vi "FGV_REPORTS_records_display.vi"(7 "options":T1, 8 "error_in":errorcluster, 11 "input":variant) -> (0 "error_out":errorcluster, 3 "output":variant)   [LabVIEW 2019]
uses:
  FGV_REPORTS_records_display.ctl
  REPORTS_references.ctl
  REPORTS_all_info.ctl
  MAIN/REPORTS/GEAR/typedef/REPORT_GEAR_all_info.ctl
  MAIN/REPORTS/GEAR/typedef/REPORT_GEAR_header_data_display.ctl
  MAIN/REPORTS/GEAR/typedef/REPORT_GEAR_statuses.ctl
  MAIN/REPORTS/DATES/typedef/REPORT_DATES_all_info.ctl
  MAIN/REPORTS/DATES/typedef/REPORT_DATES_statuses.ctl
  MAIN/REPORTS/PRODUCTION_BATCH/typedef/REPORT_PBATCH_all_info.ctl
  MAIN/REPORTS/OPERATION/typedef/REPORT_OPRTN_all_info.ctl
  MAIN/REPORTS/CONFIG_HISTORY/typedef/REPORT_CFG_all_info.ctl
  MAIN/REPORTS/CONFIG_HISTORY/typedef/REPORT_CFG_types.ctl
  MAIN/REPORTS/AUDIT/typedef/REPORT_AUDIT_all_info.ctl
  MAIN/REPORTS/OK_NOK_COUNT/typedef/REPORT_OKNOK_all_info.ctl
  MAIN/REPORTS/REWORKS/typedef/REPORT_REWORKS_all_info.ctl
  MAIN/REPORTS/PACE/typedef/REPORT_PACE_all_info.ctl
  MAIN/REPORTS/CUSTOMER_BATCH/typedef/REPORT_CBATCH_all_info.ctl
  MAIN/REPORTS/GEAR_COMPONENTS/typedef/REPORT_CMPNT_all_info.ctl
  MAIN/REPORTS/DATES/typedef/REPORT_DATES_filters.ctl
  MAIN/REPORTS/PRODUCTION_BATCH/typedef/REPORT_PBATCH_filters.ctl
  MAIN/REPORTS/OPERATION/typedef/REPORT_OPRTN_filters.ctl
  MAIN/REPORTS/CONFIG_HISTORY/typedef/REPORT_CFG_filters.ctl
  MAIN/REPORTS/AUDIT/typedef/REPORT_AUDIT_filters.ctl
  MAIN/REPORTS/REWORKS/typedef/REPORT_REWORKS_stations.ctl
  MAIN/REPORTS/REPORT_page_change.ctl
  _misc/AULocalize/SubVIs/Get Localized Phrase Compact Interface 0D.vi
  _misc/AULocalize/SubVIs/Get Localized Phrase Compact Interface 1D.vi
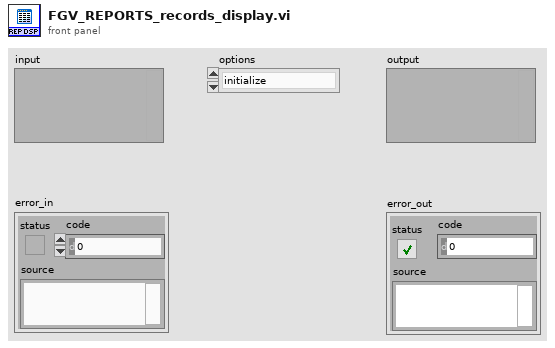
[diagram p1: front panel]
types:
  T1 = typedef "FGV_REPORTS_records_display.ctl" = enum16{"initialize", "GEAR_set_serial", "GEAR_set_header", "GEAR_set_operations", "GEAR_set_results", "GEAR_set_batches", "GEAR_get_serial", "GEAR_get_operation_IDs", "GEAR_toggle_results", "GEAR_show_all_results", "GEAR_hide_all_results", "GEAR_display", "GEAR_filter", "GEAR_restore", "GEAR_clear", "GEAR_get_all_info", "DATES_set_dates", "DATES_set_gears", "DATES_display", "DATES_filter", "DATES_first_page", "DATES_previous_page", "DATES_next_page", "DATES_last_page", "DATES_restore", "DATES_clear", "DATES_get_all_info", "PBATCH_set_batch_no", "PBATCH_set_gears", "PBATCH_display", "PBATCH_filter", "PBATCH_first_page", "PBATCH_previous_page", "PBATCH_next_page", "PBATCH_last_page", "PBATCH_restore", "PBATCH_clear", "PBATCH_get_all_info", "OPRTN_set_OP", "OPRTN_set_dates", "OPRTN_set_gears", "OPRTN_set_hidden_columns", "OPRTN_display", "OPRTN_filter", "OPRTN_filter_no_page_reset", "OPRTN_first_page", "OPRTN_previous_page", "OPRTN_next_page", "OPRTN_last_page", "OPRTN_restore", "OPRTN_clear", "OPRTN_get_all_info", "CFG_set_type", "CFG_set_dates", "CFG_set_records", "CFG_display", "CFG_filter", "CFG_first_page", "CFG_previous_page", "CFG_next_page", "CFG_last_page", "CFG_restore", "CFG_clear", "CFG_get_all_info", "AUDIT_set_dates", "AUDIT_set_records", "AUDIT_display", "AUDIT_filter", "AUDIT_first_page", "AUDIT_previous_page", "AUDIT_next_page", "AUDIT_last_page", "AUDIT_restore", "AUDIT_clear", "AUDIT_get_all_info", "OKNOK_set_dates", "OKNOK_set_records", "OKNOK_display", "OKNOK_restore", "OKNOK_clear", "OKNOK_get_all_info", "REWORKS_set_dates", "REWORKS_set_from_to", "REWORKS_set_records", "REWORKS_display", "REWORKS_filter", "REWORKS_first_page", "REWORKS_previous_page", "REWORKS_next_page", "REWORKS_last_page", "REWORKS_restore", "REWORKS_clear", "REWORKS_get_all_info", "PACE_set_dates", "PACE_set_limits", "PACE_set_records", "PACE_display", "PACE_restore", "PACE_clear", "PACE_get_all_info", "CBATCH_set_code", "CBATCH_set_records", "CBATCH_display", "CBATCH_filter", "CBATCH_first_page", "CBATCH_previous_page", "CBATCH_next_page", "CBATCH_last_page", "CBATCH_restore", "CBATCH_clear", "CBATCH_get_all_info", "CMPNT_set_serial", "CMPNT_set_records", "CMPNT_display", "CMPNT_first_page", "CMPNT_previous_page", "CMPNT_next_page", "CMPNT_last_page", "CMPNT_restore", "CMPNT_clear", "CMPNT_get_all_info", "clear"}
  T2 = typedef "REPORTS_all_info.ctl" = cluster{"REPORT_GEAR_all_info":T3, "REPORT_DATES_all_info":T6, "REPORT_PBATCH_all_info":T8, "REPORT_OPRTN_all_info":T9, "REPORT_CFG_all_info":T10, "REPORT_AUDIT_all_info":T12, "REPORT_OKNOK_all_info":T13, "REPORT_REWORKS_all_info":T14, "REPORT_PACE_all_info":T15, "REPORT_CBATCH_all_info":T16, "REPORT_CMPNT_all_info":T17, "REPORTS_references":T18}
  T3 = typedef "REPORT_GEAR_all_info.ctl" = cluster{"serial":string, "filter_OP":string, "REPORT_GEAR_header":T4, "operations":string[][], "operation_statuses":T5[], "results":string[][], "result_statuses":T5[], "batches":string[][], "batch_statuses":T5[], "column_headers":string[], "displayed_rows":string[][], "displayed_statuses":T5[], "column_widths":i16[]}
  T4 = typedef "REPORT_GEAR_header_data_display.ctl" = cluster{"ID":string, "creation_time":string, "last_station":string, "last_status":string, "pinion_serial":string, "batch_code":string}
  T5 = typedef "REPORT_GEAR_statuses.ctl" = enum16{"OP_OK_hide", "OP_OK_show", "OP_NOK_hide", "OP_NOK_show", "OP_interrupted_hide", "OP_interrupted_show", "OP_in_operation_hide", "OP_in_operation_show", "OP_unexpected_hide", "OP_unexpected_show", "RE_REAL_OK", "RE_REAL_NOK", "RE_STRING", "RE_sub_header", "RE_no_data", "RE_unexpected", "BA_sub_header", "BA_data", "BA_no_data"}
  T6 = typedef "REPORT_DATES_all_info.ctl" = cluster{"date_start":string, "date_end":string, "time_start":string, "time_end":string, "filter_last_OP":string, "filter_last_status":string, "gears":string[][], "gears_statuses":T7[], "column_headers":string[], "displayed_rows":string[][], "displayed_statuses":T7[], "column_widths":i16[], "active_page":i32}
  T7 = typedef "REPORT_DATES_statuses.ctl" = enum16{"GEAR_OK", "GEAR_NOK", "GEAR_interrupted", "GEAR_in_operation", "GEAR_unexpected"}
  T8 = typedef "REPORT_PBATCH_all_info.ctl" = cluster{"batch_no":string, "filter_last_OP":string, "filter_last_status":string, "gears":string[][], "gears_statuses":T7[], "column_headers":string[], "displayed_rows":string[][], "displayed_statuses":T7[], "column_widths":i16[], "active_page":i32}
  T9 = typedef "REPORT_OPRTN_all_info.ctl" = cluster{"OP":string, "date_start":string, "date_end":string, "time_start":string, "time_end":string, "filter_last_status":string, "no_of_static_columns":i32, "operations":string[][], "operations_statuses":T7[], "column_headers":string[], "archivisation_description":string[][], "displayed_rows":string[][], "displayed_statuses":T7[], "column_widths":i16[], "hidden_columns":i32[], "active_page":i32}
  T10 = typedef "REPORT_CFG_all_info.ctl" = cluster{"type":T11, "date_start":string, "date_end":string, "time_start":string, "time_end":string, "filter_OP":string, "records":string[][], "column_headers":string[], "displayed_rows":string[][], "column_widths":i16[], "active_page":i32}
  T11 = typedef "REPORT_CFG_types.ctl" = enum16{"REFERENCE", "ARCHIVISATION", "USERS"}
  T12 = typedef "REPORT_AUDIT_all_info.ctl" = cluster{"date_start":string, "date_end":string, "time_start":string, "time_end":string, "filter_OP":string, "filter_status":string, "records":string[][], "record_statuses":T7[], "column_headers":string[], "displayed_rows":string[][], "displayed_statuses":T7[], "column_widths":i16[], "active_page":i32}
  T13 = typedef "REPORT_OKNOK_all_info.ctl" = cluster{"date_start":string, "date_end":string, "time_start":string, "time_end":string, "records":string[][], "column_headers":string[], "column_widths":i16[]}
  T14 = typedef "REPORT_REWORKS_all_info.ctl" = cluster{"date_start":string, "date_end":string, "time_start":string, "time_end":string, "from_OP":string, "to_OP":string, "records":string[][], "record_statuses":T7[], "column_headers":string[], "displayed_rows":string[][], "displayed_statuses":T7[], "column_widths":i16[], "active_page":i32}
  T15 = typedef "REPORT_PACE_all_info.ctl" = cluster{"date_start":string, "date_end":string, "time_start":string, "time_end":string, "low_limit":u16, "high_limit":u16, "records":string[][], "column_headers":string[], "column_widths":i16[]}
  T16 = typedef "REPORT_CBATCH_all_info.ctl" = cluster{"batch_code":string, "records":string[][], "record_statuses":T7[], "column_headers":string[], "displayed_rows":string[][], "displayed_statuses":T7[], "column_widths":i16[], "active_page":i32}
  T17 = typedef "REPORT_CMPNT_all_info.ctl" = cluster{"gear_serial":string, "records":string[][], "column_headers":string[], "displayed_rows":string[][], "column_widths":i16[], "active_page":i32}
  T18 = typedef "REPORTS_references.ctl" = cluster{"front_panel_reference":refnum<vi>, "SQL_listbox_reference":refnum<vi>, "REPORT_page_first":refnum<vi>, "REPORT_page_previous":refnum<vi>, "REPORT_page_next":refnum<vi>, "REPORT_page_last":refnum<vi>, "REPORT_page_counter":refnum<vi>, "REPORT_GEAR_serial":refnum<vi>, "REPORT_GEAR_serial_display":refnum<vi>, "REPORT_GEAR_station":refnum<vi>, "REPORT_GEAR_header_data_display":refnum<vi>, "REPORT_DATES_start":refnum<vi>, "REPORT_DATES_end":refnum<vi>, "REPORT_DATES_time_start":refnum<vi>, "REPORT_DATES_time_end":refnum<vi>, "REPORT_DATES_order_selection":refnum<vi>, "REPORT_DATES_last_OP":refnum<vi>, "REPORT_DATES_last_status":refnum<vi>, "REPORT_PBATCH_batch_no":refnum<vi>, "REPORT_PBATCH_order_selection":refnum<vi>, "REPORT_PBATCH_last_op":refnum<vi>, "REPORT_PBATCH_last_status":refnum<vi>, "REPORT_OPRTN_operation":refnum<vi>, "REPORT_OPRTN_start":refnum<vi>, "REPORT_OPRTN_end":refnum<vi>, "REPORT_OPRTN_time_start":refnum<vi>, "REPORT_OPRTN_time_end":refnum<vi>, "REPORT_OPRTN_order_selection":refnum<vi>, "REPORT_OPRTN_last_status":refnum<vi>, "REPORT_CFG_type":refnum<vi>, "REPORT_CFG_start":refnum<vi>, "REPORT_CFG_end":refnum<vi>, "REPORT_CFG_time_start":refnum<vi>, "REPORT_CFG_time_end":refnum<vi>, "REPORT_CFG_order_selection":refnum<vi>, "REPORT_CFG_op_filter":refnum<vi>, "REPORT_AUDIT_start":refnum<vi>, "REPORT_AUDIT_end":refnum<vi>, "REPORT_AUDIT_time_start":refnum<vi>, "REPORT_AUDIT_time_end":refnum<vi>, "REPORT_AUDIT_order_selection":refnum<vi>, "REPORT_AUDIT_op_filter":refnum<vi>, "REPORT_AUDIT_status_filter":refnum<vi>, "REPORT_OKNOK_start":refnum<vi>, "REPORT_OKNOK_end":refnum<vi>, "REPORT_OKNOK_time_start":refnum<vi>, "REPORT_OKNOK_time_end":refnum<vi>, "REPORT_REWORKS_start":refnum<vi>, "REPORT_REWORKS_end":refnum<vi>, "REPORT_REWORKS_time_start":refnum<vi>, "REPORT_REWORKS_time_end":refnum<vi>, "REPORT_REWORKS_from_OP":refnum<vi>, "REPORT_REWORKS_to_OP":refnum<vi>, "REPORT_REWORKS_order_selection":refnum<vi>, "REPORT_PACE_start":refnum<vi>, "REPORT_PACE_end":refnum<vi>, "REPORT_PACE_time_start":refnum<vi>, "REPORT_PACE_time_end":refnum<vi>, "REPORT_PACE_low_limit":refnum<vi>, "REPORT_PACE_high_limit":refnum<vi>, "REPORT_CBATCH_batch_code":refnum<vi>, "REPORT_CBATCH_order_selection":refnum<vi>, "REPORT_CMPNT_gear_serial":refnum<vi>}
  T19 = typedef "REPORT_DATES_filters.ctl" = cluster{"order_selection":enum32{"old_to_new", "new_to_old"}, "last_OP":string, "last_status":string}
  T20 = typedef "REPORT_page_change.ctl" = enum16{"first", "previous", "next", "last"}
  T21 = typedef "REPORT_PBATCH_filters.ctl" = cluster{"order_selection":enum32{"old_to_new", "new_to_old"}, "last_OP":string, "last_status":string}
  T22 = typedef "REPORT_OPRTN_filters.ctl" = cluster{"order_selection":enum32{"old_to_new", "new_to_old"}, "last_status":string}
  T23 = typedef "REPORT_CFG_filters.ctl" = cluster{"order_selection":enum32{"old_to_new", "new_to_old"}, "OP":string}
  T24 = typedef "REPORT_AUDIT_filters.ctl" = cluster{"order_selection":enum32{"old_to_new", "new_to_old"}, "OP_filter":string, "status_filter":string}
  T25 = typedef "REPORT_REWORKS_stations.ctl" = u16
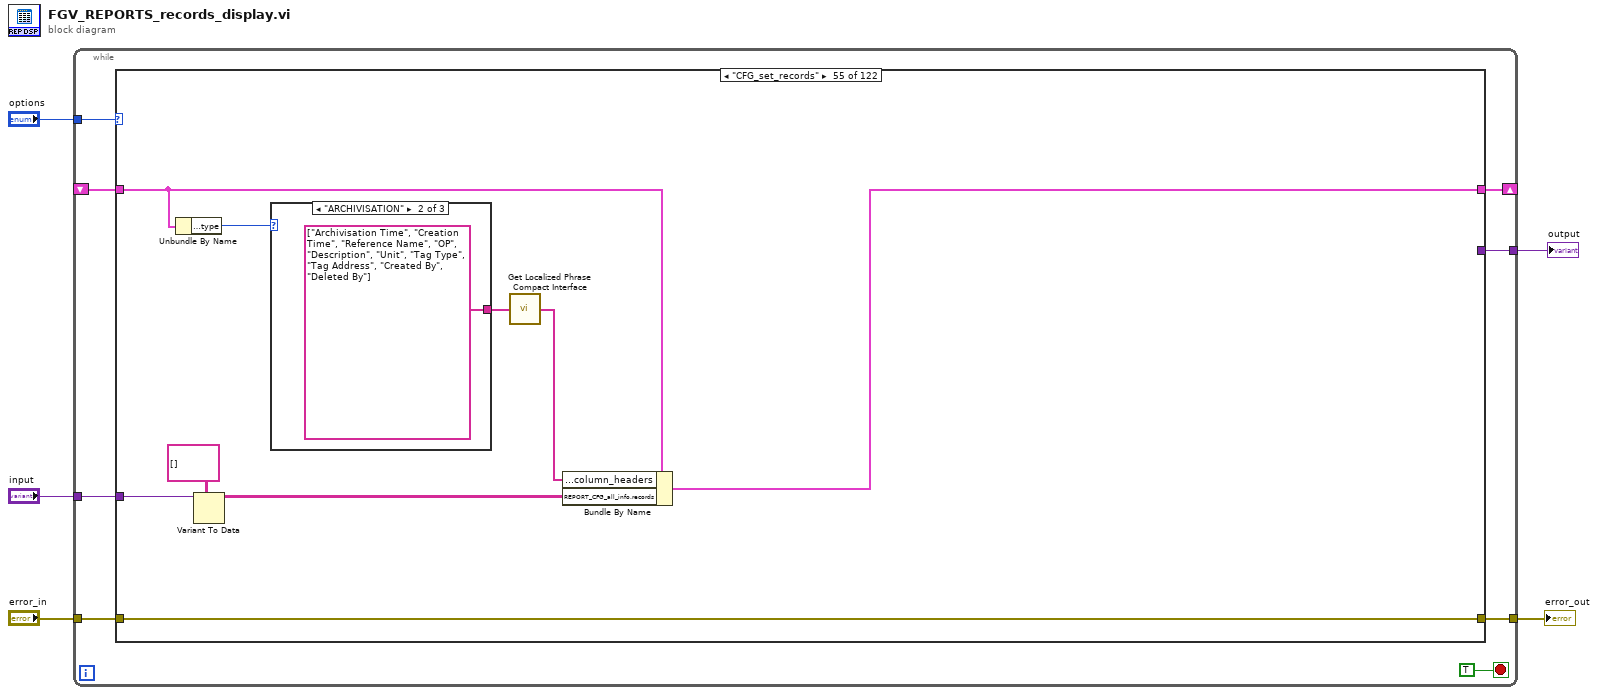
[diagram p0: block diagram]
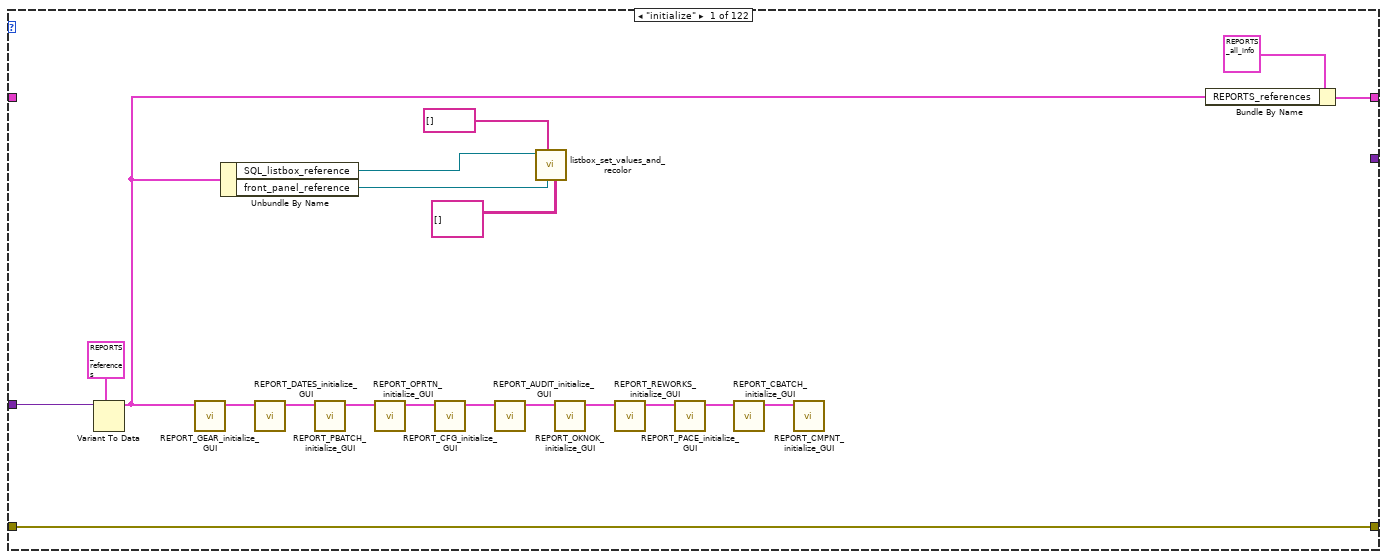
[diagram p2: hidden frame]
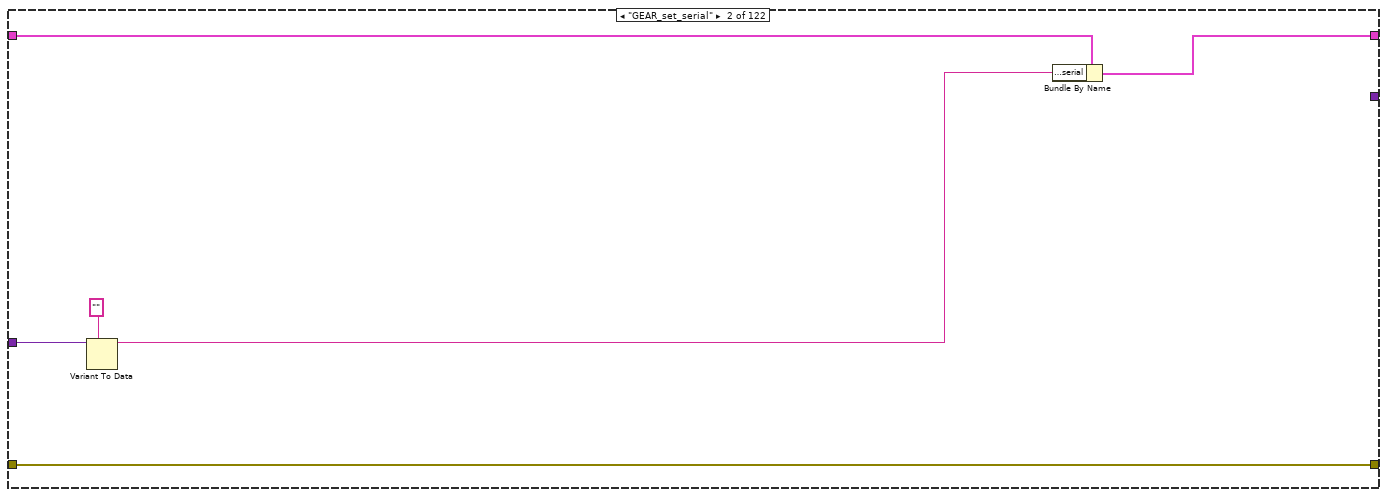
[diagram p3: hidden frame]
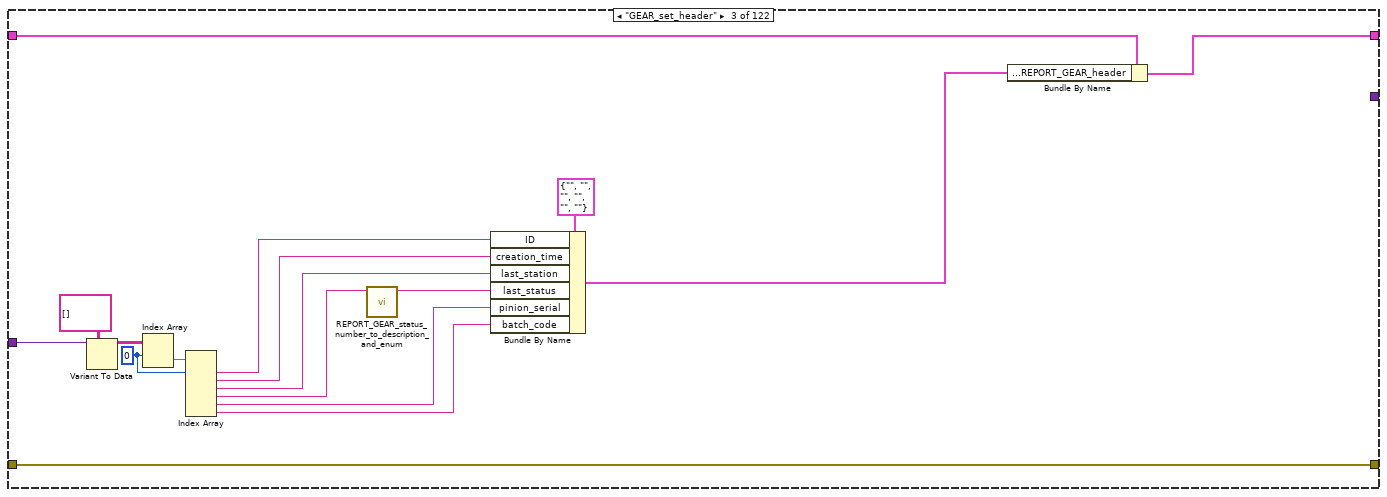
[diagram p4: hidden frame]
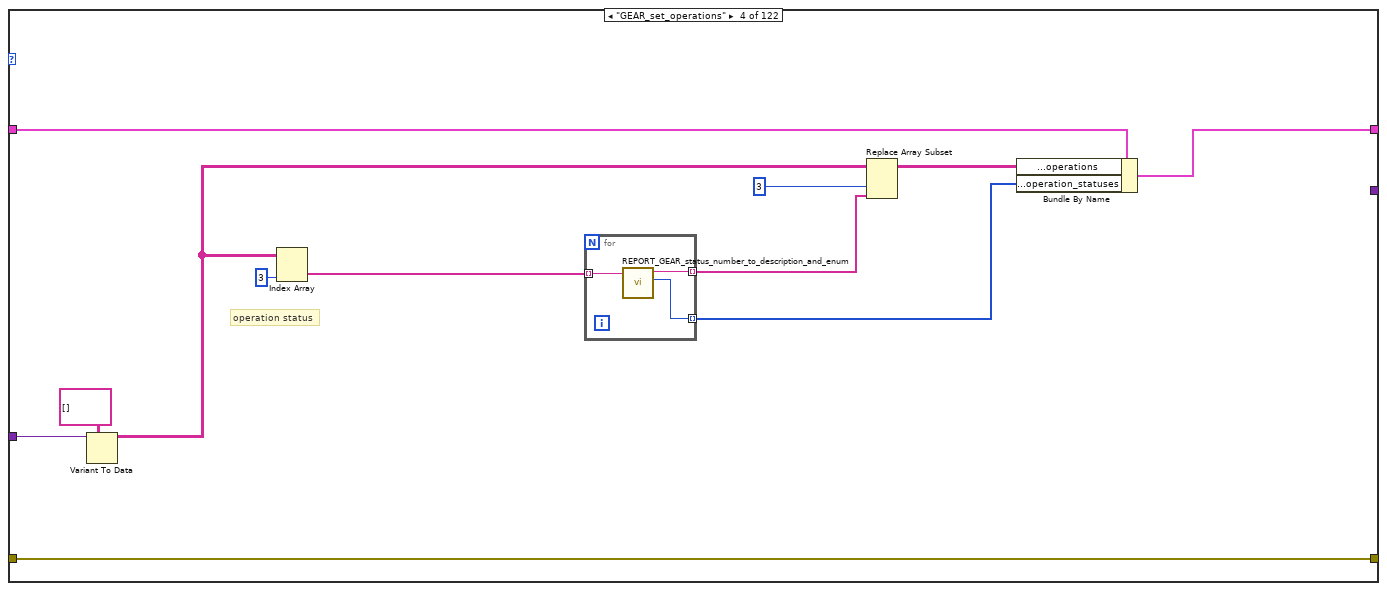
[diagram p5: hidden frame]
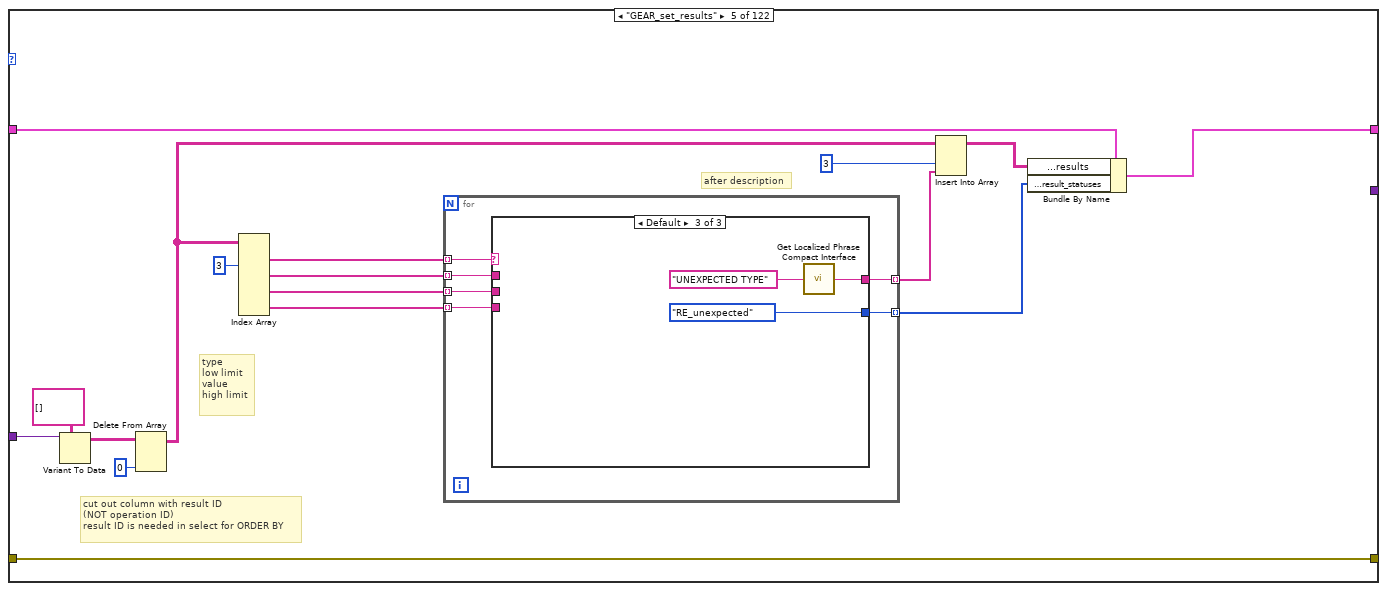
[diagram p6: hidden frame]
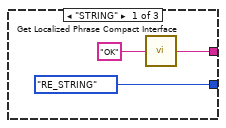
[diagram p7: hidden frame]
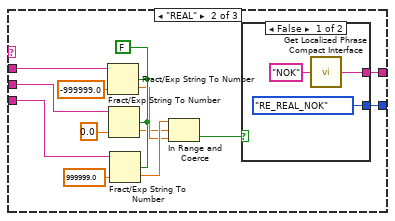
[diagram p8: hidden frame]
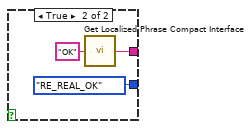
[diagram p9: hidden frame]
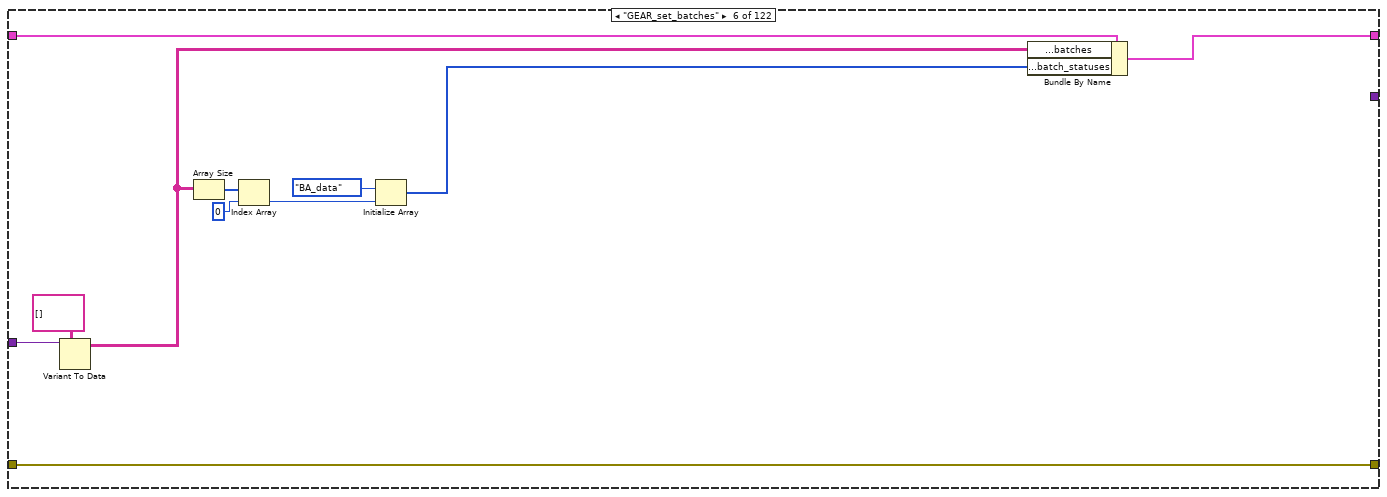
[diagram p10: hidden frame]
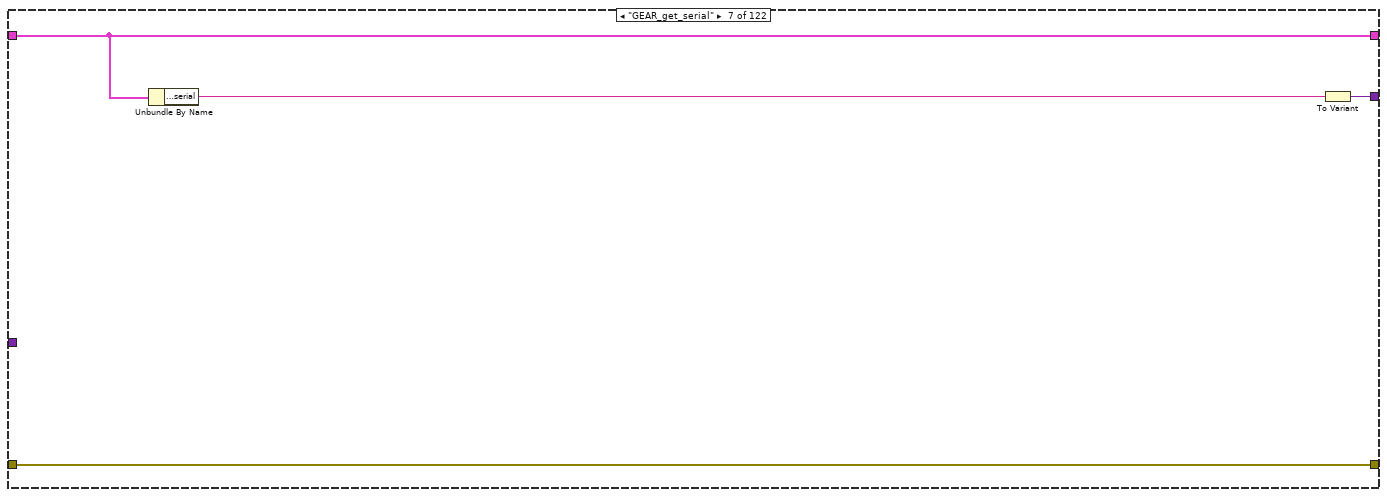
[diagram p11: hidden frame]
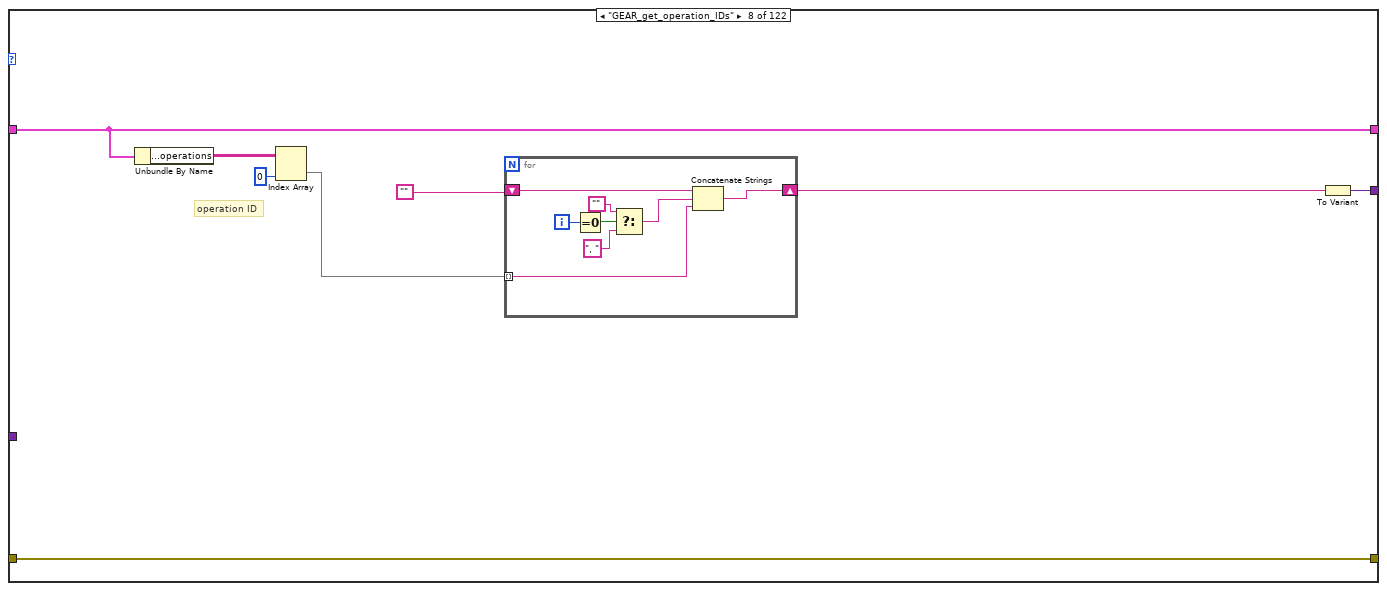
[diagram p12: hidden frame]
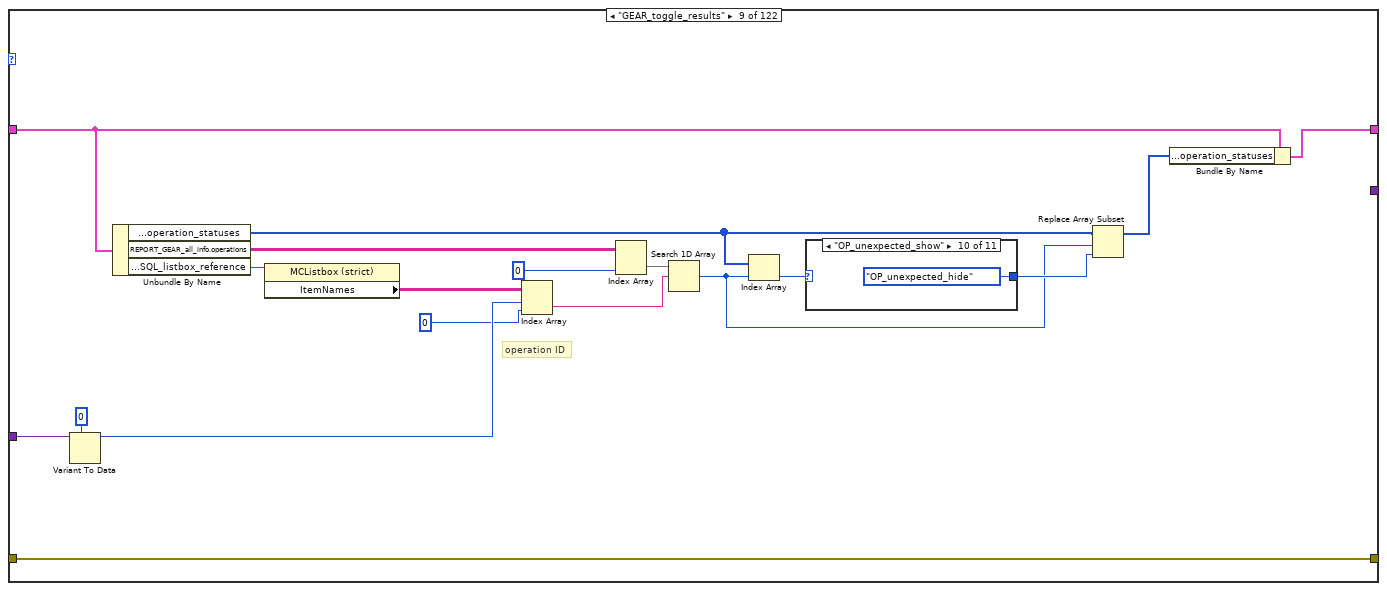
[diagram p13: hidden frame]
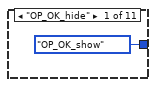
[diagram p14: hidden frame]
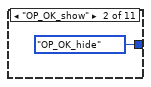
[diagram p15: hidden frame]
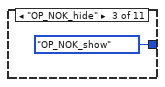
[diagram p16: hidden frame]
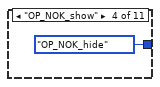
[diagram p17: hidden frame]
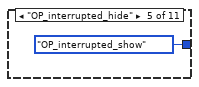
[diagram p18: hidden frame]
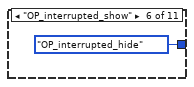
[diagram p19: hidden frame]
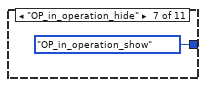
[diagram p20: hidden frame]
diagram:
  n1 = while {
    tunnel: "options" -> [w12]
    tunnel: [w11] -> w5
    tunnel: "error_in" -> [w10]
    shift-right: [w9] -> _
    shift-left: _ -> [w8]
    tunnel: "input" -> [w7]
    tunnel: [w6] -> w1
    stop <- TRUE stop-if-true
    n2 = case shown="\"CFG_set_records\"" w12 {
      tunnel: [w33 w39 w56 w68 w88 w130 w134 w142 w168 w184 w197 w212 w218 w220 w229 w233 w244 w256 w269 w275 w279 w283 w287 w291 w293 w302 w306 w312 w324 w337 w343 w347 w351 w355 w359 w361 w370 w374 w380 w391 w410 w425 w434 w441 w448 w452 w456 w460 w464 w466 w475 w479 w485 w496 w505 w516 w522 w526 w530 w534 w538 w540 w549 w553 w564 w576 w589 w595 w599 w603 w607 w611 w613 w622 w626 w637 w643 w648 w650 w659 w663 w674 w683 w695 w706 w712 w716 w720 w724 w728 w730 w739 w743 w754 w762 w768 w773 w775 w784 w788 w794 w806 w817 w823 w827 w831 w835 w839 w841 w850 w854 w860 w866 w871 w875 w879 w883 w887 w889 w898 w902 w911] -> w11
      tunnel: w10 -> [w33 w39 w56 w68 w88 w130 w134 w142 w168 w184 w197 w212 w218 w220 w229 w233 w244 w256 w269 w275 w279 w283 w287 w291 w293 w302 w306 w312 w324 w337 w343 w347 w351 w355 w359 w361 w370 w374 w380 w391 w410 w425 w434 w441 w448 w452 w456 w460 w464 w466 w475 w479 w485 w496 w505 w516 w522 w526 w530 w534 w538 w540 w549 w553 w564 w576 w589 w595 w599 w603 w607 w611 w613 w622 w626 w637 w643 w648 w650 w659 w663 w674 w683 w695 w706 w712 w716 w720 w724 w728 w730 w739 w743 w754 w762 w768 w773 w775 w784 w788 w794 w806 w817 w823 w827 w831 w835 w839 w841 w850 w854 w860 w866 w871 w875 w879 w883 w887 w889 w898 w902 w911]
      tunnel: [w25 w38 w55 w67 w87 w129 w132 w140 w152 w182 w195 w207 w217 w219 w228 w232 w238 w255 w262 w274 w277 w281 w285 w289 w292 w301 w305 w311 w323 w330 w340 w345 w349 w353 w357 w360 w369 w373 w379 w385 w409 w422 w428 w438 w445 w450 w454 w458 w462 w465 w474 w478 w484 w490 w503 w510 w519 w524 w528 w532 w536 w539 w548 w552 w558 w575 w582 w594 w597 w601 w605 w609 w612 w621 w625 w631 w642 w645 w649 w658 w662 w668 w682 w694 w700 w711 w714 w718 w722 w726 w729 w738 w742 w748 w761 w767 w770 w774 w783 w787 w791 w805 w812 w822 w825 w829 w833 w837 w840 w849 w853 w857 w865 w868 w873 w877 w881 w885 w888 w897 w901 w903] -> w9
      tunnel: w8 -> [_ w36 w53 w65 w85 w127 w132 w140 w153 w183 w196 w208 w216 w219 w227 w232 w239 w253 w267 w273 w278 w282 w286 w290 w292 w300 w305 w309 w321 w335 w341 w346 w350 w354 w358 w360 w368 w373 w377 w386 w407 w423 w433 w439 w446 w451 w455 w459 w463 w465 w473 w478 w482 w491 w500 w515 w520 w525 w529 w533 w537 w539 w547 w552 w559 w573 w587 w593 w598 w602 w606 w610 w612 w620 w625 w632 w640 w646 w649 w657 w662 w669 w680 w692 w704 w710 w715 w719 w723 w727 w729 w737 w742 w749 w759 w765 w771 w774 w782 w787 w792 w803 w815 w821 w826 w830 w834 w838 w840 w848 w853 w858 w863 w869 w874 w878 w882 w886 w888 w896 w901 w908]
      tunnel: w7 -> [w29 w37 w54 w66 w86 w128 _ _ w166 _ _ _ w215 _ _ _ w243 w254 w266 w272 _ _ _ _ _ _ _ w310 w322 w334 w342 _ _ _ _ _ _ _ w378 w390 w408 w424 w432 w440 w447 _ _ _ _ _ _ _ w483 w495 w504 w514 w521 _ _ _ _ _ _ _ w563 w574 w586 w592 _ _ _ _ _ _ _ w636 w641 _ _ _ _ w673 w681 w693 w703 w709 _ _ _ _ _ _ _ w753 w760 w766 _ _ _ _ w793 w804 w814 w820 _ _ _ _ _ _ _ w859 w864 _ _ _ _ _ _ _ _ _]
      tunnel: [_ _ _ _ _ _ w133 w141 _ _ _ _ _ _ _ w230 _ _ _ _ _ _ _ _ _ _ w303 _ _ _ _ _ _ _ _ _ _ w371 _ _ _ _ _ _ _ _ _ _ _ _ _ w476 _ _ _ _ _ _ _ _ _ _ _ w550 _ _ _ _ _ _ _ _ _ _ w623 _ _ _ _ _ w660 _ _ _ _ _ _ _ _ _ _ _ w740 _ _ _ _ _ _ w785 _ _ _ _ _ _ _ _ _ _ w851 _ _ _ _ _ _ _ _ _ w899 _] -> w6
      frame "initialize" {
        n3 = Variant To Data(type=T18 {"front_panel_reference"=refnum, "SQL_listbox_reference"=refnum, "REPORT_page_first"=refnum, "REPORT_page_previous"=refnum, "REPORT_page_next"=refnum, "REPORT_page_last"=refnum, "REPORT_page_counter"=refnum, "REPORT_GEAR_serial"=refnum, "REPORT_GEAR_serial_display"=refnum, "REPORT_GEAR_station"=refnum, "REPORT_GEAR_header_data_display"=refnum, "REPORT_DATES_start"=refnum, "REPORT_DATES_end"=refnum, "REPORT_DATES_time_start"=refnum, "REPORT_DATES_time_end"=refnum, "REPORT_DATES_order_selection"=refnum, "REPORT_DATES_last_OP"=refnum, "REPORT_DATES_last_status"=refnum, "REPORT_PBATCH_batch_no"=refnum, "REPORT_PBATCH_order_selection"=refnum, "REPORT_PBATCH_last_op"=refnum, "REPORT_PBATCH_last_status"=refnum, "REPORT_OPRTN_operation"=refnum, "REPORT_OPRTN_start"=refnum, "REPORT_OPRTN_end"=refnum, "REPORT_OPRTN_time_start"=refnum, "REPORT_OPRTN_time_end"=refnum, "REPORT_OPRTN_order_selection"=refnum, "REPORT_OPRTN_last_status"=refnum, "REPORT_CFG_type"=refnum, "REPORT_CFG_start"=refnum, "REPORT_CFG_end"=refnum, "REPORT_CFG_time_start"=refnum, "REPORT_CFG_time_end"=refnum, "REPORT_CFG_order_selection"=refnum, "REPORT_CFG_op_filter"=refnum, "REPORT_AUDIT_start"=refnum, "REPORT_AUDIT_end"=refnum, "REPORT_AUDIT_time_start"=refnum, "REPORT_AUDIT_time_end"=refnum, "REPORT_AUDIT_order_selection"=refnum, "REPORT_AUDIT_op_filter"=refnum, "REPORT_AUDIT_status_filter"=refnum, "REPORT_OKNOK_start"=refnum, "REPORT_OKNOK_end"=refnum, "REPORT_OKNOK_time_start"=refnum, "REPORT_OKNOK_time_end"=refnum, "REPORT_REWORKS_start"=refnum, "REPORT_REWORKS_end"=refnum, "REPORT_REWORKS_time_start"=refnum, "REPORT_REWORKS_time_end"=refnum, "REPORT_REWORKS_from_OP"=refnum, "REPORT_REWORKS_to_OP"=refnum, "REPORT_REWORKS_order_selection"=refnum, "REPORT_PACE_start"=refnum, "REPORT_PACE_end"=refnum, "REPORT_PACE_time_start"=refnum, "REPORT_PACE_time_end"=refnum, "REPORT_PACE_low_limit"=refnum, "REPORT_PACE_high_limit"=refnum, "REPORT_CBATCH_batch_code"=refnum, "REPORT_CBATCH_order_selection"=refnum, "REPORT_CMPNT_gear_serial"=refnum} ("REPORTS_references"), Variant=w29) -> (data=w24:T18)  [unwired: 1 in, 1 out]
        n4 = call "REPORT_GEAR_initialize_GUI.vi"("REPORTS_references_in"=w24) -> ("REPORTS_references_out"=w23:T18)  [unwired: 10 in]
        n5 = Unbundle By Name(w24) -> ("SQL_listbox_reference"=w27:refnum<vi>, "front_panel_reference"=w28:refnum<vi>)
        n6 = call "REPORT_DATES_initialize_GUI.vi"("REPORTS_references_in"=w23) -> ("REPORTS_references_out"=w22:T18)  [unwired: 10 in]
        n7 = call "REPORT_PBATCH_initialize_GUI.vi"("REPORTS_references_in"=w22) -> ("REPORTS_references_out"=w21:T18)  [unwired: 10 in]
        n8 = call "REPORT_OPRTN_initialize_GUI.vi"("REPORTS_references_in"=w21) -> ("REPORTS_references_out"=w20:T18)  [unwired: 10 in]
        n9 = call "REPORT_CFG_initialize_GUI.vi"("REPORTS_references_in"=w20) -> ("REPORTS_references_out"=w19:T18)  [unwired: 10 in]
        n10 = call "REPORT_AUDIT_initialize_GUI.vi"("REPORTS_references_in"=w19) -> ("REPORTS_references_out"=w18:T18)  [unwired: 10 in]
        n11 = call "listbox_set_values_and_recolor.vi"("item_names"=string[][] [], "front_panel_reference"=w28, "column_names"=string[] [], "multicolumn_listbox_reference_in"=w27) -> ()  [unwired: 6 in, 2 out]
        n12 = call "REPORT_OKNOK_initialize_GUI.vi"("REPORTS_references_in"=w18) -> ("REPORTS_references_out"=w17:T18)  [unwired: 10 in]
        n13 = call "REPORT_REWORKS_initialize_GUI.vi"("REPORTS_references_in"=w17) -> ("REPORTS_references_out"=w16:T18)  [unwired: 10 in]
        n14 = call "REPORT_PACE_initialize_GUI.vi"("REPORTS_references_in"=w16) -> ("REPORTS_references_out"=w15:T18)  [unwired: 10 in]
        n15 = call "REPORT_CBATCH_initialize_GUI.vi"("REPORTS_references_in"=w15) -> ("REPORTS_references_out"=w14:T18)  [unwired: 10 in]
        n16 = call "REPORT_CMPNT_initialize_GUI.vi"("REPORTS_references_in"=w14) -> ()  [unwired: 10 in, 1 out]
        n17 = Bundle By Name(cluster=T2 {"REPORT_GEAR_all_info"={"serial"="", "filter_OP"="", "REPORT_GEAR_header"={"ID"="", "creation_time"="", "last_station"="", "last_status"="", "pinion_serial"="", "batch_code"=""}, "operations"=[], "operation_statuses"=[], "results"=[], "result_statuses"=[], "batches"=[], "batch_statuses"=[], "column_headers"=[], "displayed_rows"=[], "displayed_statuses"=[], "column_widths"=[]}, "REPORT_DATES_all_info"={"date_start"="", "date_end"="", "time_start"="", "time_end"="", "filter_last_OP"="", "filter_last_status"="", "gears"=[], "gears_statuses"=[], "column_headers"=[], "displayed_rows"=[], "displayed_statuses"=[], "column_widths"=[], "active_page"=0}, "REPORT_PBATCH_all_info"={"batch_no"="", "filter_last_OP"="", "filter_last_status"="", "gears"=[], "gears_statuses"=[], "column_headers"=[], "displayed_rows"=[], "displayed_statuses"=[], "column_widths"=[], "active_page"=0}, "REPORT_OPRTN_all_info"={"OP"="", "date_start"="", "date_end"="", "time_start"="", "time_end"="", "filter_last_status"="", "no_of_static_columns"=0, "operations"=[], "operations_statuses"=[], "column_headers"=[], "archivisation_description"=[], "displayed_rows"=[], "displayed_statuses"=[], "column_widths"=[], "hidden_columns"=[], "active_page"=0}, "REPORT_CFG_all_info"={"type"=enum."REFERENCE", "date_start"="", "date_end"="", "time_start"="", "time_end"="", "filter_OP"="", "records"=[], "column_headers"=[], "displayed_rows"=[], "column_widths"=[], "active_page"=0}, "REPORT_AUDIT_all_info"={"date_start"="", "date_end"="", "time_start"="", "time_end"="", "filter_OP"="", "filter_status"="", "records"=[], "record_statuses"=[], "column_headers"=[], "displayed_rows"=[], "displayed_statuses"=[], "column_widths"=[], "active_page"=0}, "REPORT_OKNOK_all_info"={"date_start"="", "date_end"="", "time_start"="", "time_end"="", "records"=[], "column_headers"=[], "column_widths"=[]}, "REPORT_REWORKS_all_info"={"date_start"="", "date_end"="", "time_start"="", "time_end"="", "from_OP"="", "to_OP"="", "records"=[], "record_statuses"=[], "column_headers"=[], "displayed_rows"=[], "displayed_statuses"=[], "column_widths"=[], "active_page"=0}, "REPORT_PACE_all_info"={"date_start"="", "date_end"="", "time_start"="", "time_end"="", "low_limit"=0, "high_limit"=0, "records"=[], "column_headers"=[], "column_widths"=[]}, "REPORT_CBATCH_all_info"={"batch_code"="", "records"=[], "record_statuses"=[], "column_headers"=[], "displayed_rows"=[], "displayed_statuses"=[], "column_widths"=[], "active_page"=0}, "REPORT_CMPNT_all_info"={"gear_serial"="", "records"=[], "column_headers"=[], "displayed_rows"=[], "column_widths"=[], "active_page"=0}, "REPORTS_references"={"front_panel_reference"=refnum, "SQL_listbox_reference"=refnum, "REPORT_page_first"=refnum, "REPORT_page_previous"=refnum, "REPORT_page_next"=refnum, "REPORT_page_last"=refnum, "REPORT_page_counter"=refnum, "REPORT_GEAR_serial"=refnum, "REPORT_GEAR_serial_display"=refnum, "REPORT_GEAR_station"=refnum, "REPORT_GEAR_header_data_display"=refnum, "REPORT_DATES_start"=refnum, "REPORT_DATES_end"=refnum, "REPORT_DATES_time_start"=refnum, "REPORT_DATES_time_end"=refnum, "REPORT_DATES_order_selection"=refnum, "REPORT_DATES_last_OP"=refnum, "REPORT_DATES_last_status"=refnum, "REPORT_PBATCH_batch_no"=refnum, "REPORT_PBATCH_order_selection"=refnum, "REPORT_PBATCH_last_op"=refnum, "REPORT_PBATCH_last_status"=refnum, "REPORT_OPRTN_operation"=refnum, "REPORT_OPRTN_start"=refnum, "REPORT_OPRTN_end"=refnum, "REPORT_OPRTN_time_start"=refnum, "REPORT_OPRTN_time_end"=refnum, "REPORT_OPRTN_order_selection"=refnum, "REPORT_OPRTN_last_status"=refnum, "REPORT_CFG_type"=refnum, "REPORT_CFG_start"=refnum, "REPORT_CFG_end"=refnum, "REPORT_CFG_time_start"=refnum, "REPORT_CFG_time_end"=refnum, "REPORT_CFG_order_selection"=refnum, "REPORT_CFG_op_filter"=refnum, "REPORT_AUDIT_start"=refnum, "REPORT_AUDIT_end"=refnum, "REPORT_AUDIT_time_start"=refnum, "REPORT_AUDIT_time_end"=refnum, "REPORT_AUDIT_order_selection"=refnum, "REPORT_AUDIT_op_filter"=refnum, "REPORT_AUDIT_status_filter"=refnum, "REPORT_OKNOK_start"=refnum, "REPORT_OKNOK_end"=refnum, "REPORT_OKNOK_time_start"=refnum, "REPORT_OKNOK_time_end"=refnum, "REPORT_REWORKS_start"=refnum, "REPORT_REWORKS_end"=refnum, "REPORT_REWORKS_time_start"=refnum, "REPORT_REWORKS_time_end"=refnum, "REPORT_REWORKS_from_OP"=refnum, "REPORT_REWORKS_to_OP"=refnum, "REPORT_REWORKS_order_selection"=refnum, "REPORT_PACE_start"=refnum, "REPORT_PACE_end"=refnum, "REPORT_PACE_time_start"=refnum, "REPORT_PACE_time_end"=refnum, "REPORT_PACE_low_limit"=refnum, "REPORT_PACE_high_limit"=refnum, "REPORT_CBATCH_batch_code"=refnum, "REPORT_CBATCH_order_selection"=refnum, "REPORT_CMPNT_gear_serial"=refnum}} ("REPORT_all_info"), "REPORTS_references"=w24) -> (w25:T2)
      }
      frame "GEAR_set_serial" {
        n18 = Variant To Data(type="", Variant=w37) -> (data=w34:string)  [unwired: 1 in, 1 out]
        n19 = Bundle By Name(cluster=w36, "REPORT_GEAR_all_info.serial"=w34) -> (w38:T2)
      }
      frame "GEAR_set_header" {
        w47 = 0 ("index (row)")
        n20 = Variant To Data(type=string[][] [], Variant=w54) -> (data=w49:string[][])  [unwired: 1 in, 1 out]
        n21 = Index Array(array=w49, index (row)=w47) -> (element=w48:string[])  [unwired: 1 in]
        n22 = Index Array(array=w48, index #1=w47) -> (element #1=w45:string, element #2=w46:string, element #3=w44:string, element #4=w42:string, element #5=w43:string, element #6=w40:string)  [unwired: 5 in]
        n23 = call "REPORT_GEAR_status_number_to_description_and_enum.vi"("status_nmb"=w42) -> ("status_description"=w41:string)  [unwired: 9 in, 1 out]
        n24 = Bundle By Name(cluster=T4 {"ID"="", "creation_time"="", "last_station"="", "last_status"="", "pinion_serial"="", "batch_code"=""} ("REPORT_GEAR_header_data_display"), "ID"=w45, "creation_time"=w46, "last_station"=w44, "last_status"=w41, "pinion_serial"=w43, "batch_code"=w40) -> (w50:T4)
        n25 = Bundle By Name(cluster=w53, "REPORT_GEAR_all_info.REPORT_GEAR_header"=w50) -> (w55:T2)
      }
      frame "GEAR_set_operations" {
        # "operation status"
        n26 = Variant To Data(type=string[][] [], Variant=w66) -> (data=w60:string[][])  [unwired: 1 in, 1 out]
        n27 = Index Array(array=w60, index (col)=3 ("disabled index (col)")) -> (element=w62:string[])  [unwired: 1 in]
        n28 = for {
          tunnel: w62 -> [w71] mode=indexing
          tunnel: [w70] -> w61 mode=indexing
          tunnel: [w69] -> w57 mode=indexing
          n29 = call "REPORT_GEAR_status_number_to_description_and_enum.vi"("status_nmb"=w71) -> ("status_enum"=w70:T5, "status_description"=w69:string)  [unwired: 9 in]
        }
        n30 = Replace Array Subset(array=w60, new element=w57, index (col)=3 ("disabled index (col)")) -> (w58:string[][])  [unwired: 1 in]
        n31 = Bundle By Name(cluster=w65, "REPORT_GEAR_all_info.operations"=w58, "REPORT_GEAR_all_info.operation_statuses"=w61) -> (w67:T2)
      }
      frame "GEAR_set_results" {
        # "after description"
        # "cut out column with result ID\n(NOT operation ID)\nresult ID is needed in select for ORDER BY"
        # "type\nlow limit\nvalue\nhigh limit"
        n32 = Variant To Data(type=string[][] [], Variant=w86) -> (data=w75:string[][])  [unwired: 1 in, 1 out]
        n33 = Delete From Array(array=w75, index (col)=0 ("disabled index (col)")) -> (array with subset deleted=w74:string[][])  [unwired: 2 in, 1 out]
        n34 = Index Array(array=w74, index (col) #1=3 ("disabled index (col)")) -> (element #1=w78:string[], element #2=w83:string[], element #3=w81:string[], element #4=w80:string[])  [unwired: 7 in]
        n35 = for {
          tunnel: w83 -> [w91] mode=indexing
          tunnel: [w94] -> w82 mode=indexing
          tunnel: [w93] -> w76 mode=indexing
          tunnel: w81 -> [w90] mode=indexing
          tunnel: w80 -> [w89] mode=indexing
          tunnel: w78 -> [w92] mode=indexing
          n36 = case shown="Default" w92 {
            tunnel: [REPORT_GEAR_statuses."RE_STRING" ("REPORT_GEAR_statuses") w110 REPORT_GEAR_statuses."RE_unexpected" ("REPORT_GEAR_statuses")] -> w94
            tunnel: [w95 w109 w117] -> w93
            tunnel: w91 -> [_ w108 _]
            tunnel: w90 -> [_ w106 _]
            tunnel: w89 -> [_ w105 _]
            frame "STRING" {
              n37 = call-poly "Get Localized Phrase Compact Interface.vi"("Key"="OK") -> ("Translated Phrase"=w95:string)
            }
            frame "REAL" {
              w107 = FALSE ("use system decimal point (T)")
              n38 = Fract/Exp String To Number(use system decimal point (T)=w107, string=w108, default (0 dbl)=sgl -999999.0 ("default (0 DBL)")) -> (number=w103:sgl)  [unwired: 1 in, 1 out]
              n39 = Fract/Exp String To Number(use system decimal point (T)=w107, string=w106, default (0 dbl)=sgl 0.0 ("default (0 DBL)")) -> (number=w102:sgl)  [unwired: 1 in, 1 out]
              n40 = Fract/Exp String To Number(use system decimal point (T)=w107, string=w105, default (0 dbl)=sgl 999999.0 ("default (0 DBL)")) -> (number=w104:sgl)  [unwired: 1 in, 1 out]
              n41 = In Range and Coerce(upper limit=w104, x=w102, lower limit=w103) -> (In Range?=w101:bool)  [unwired: 1 out]
              n42 = case shown="False" w101 {
                tunnel: [REPORT_GEAR_statuses."RE_REAL_NOK" ("REPORT_GEAR_statuses") REPORT_GEAR_statuses."RE_REAL_OK" ("REPORT_GEAR_statuses")] -> w110
                tunnel: [w111 w114] -> w109
                frame False {
                  n43 = call-poly "Get Localized Phrase Compact Interface.vi"("Key"="NOK") -> ("Translated Phrase"=w111:string)
                }
                frame True {
                  n44 = call-poly "Get Localized Phrase Compact Interface.vi"("Key"="OK") -> ("Translated Phrase"=w114:string)
                }
              }
            }
            frame Default {
              n45 = call-poly "Get Localized Phrase Compact Interface.vi"("Key"="UNEXPECTED TYPE") -> ("Translated Phrase"=w117:string)
            }
          }
        }
        n46 = Insert Into Array(array=w74, index (col)=3 ("disabled index (col)"), new element=w76) -> (w77:string[][])  [unwired: 1 in]
        n47 = Bundle By Name(cluster=w85, "REPORT_GEAR_all_info.results"=w77, "REPORT_GEAR_all_info.result_statuses"=w82) -> (w87:T2)
      }
      frame "GEAR_set_batches" {
        n48 = Variant To Data(type=string[][] [], Variant=w128) -> (data=w124:string[][])  [unwired: 1 in, 1 out]
        n49 = Array Size(array=w124) -> (size(s)=w123:i32[])
        n50 = Index Array(array=w123, index=0) -> (element=w121:i32)
        n51 = Initialize Array(REPORT_GEAR_statuses."BA_data" ("REPORT_GEAR_statuses"), w121) -> (w120:T5[])
        n52 = Bundle By Name(cluster=w127, "REPORT_GEAR_all_info.batches"=w124, "REPORT_GEAR_all_info.batch_statuses"=w120) -> (w129:T2)
      }
      frame "GEAR_get_serial" {
        n53 = Unbundle By Name(w132) -> ("REPORT_GEAR_all_info.serial"=w131:string)
        n54 = To Variant(anything=w131) -> (Variant=w133:variant)
      }
      frame "GEAR_get_operation_IDs" {
        # "operation ID"
        n55 = Unbundle By Name(w140) -> ("REPORT_GEAR_all_info.operations"=w139:string[][])
        n56 = Index Array(array=w139, index (col)=0 ("disabled index (col)")) -> (element=w137:string[])  [unwired: 1 in]
        n57 = for {
          tunnel: w137 -> [w143] mode=indexing
          shift-right: [w146] -> w135
          shift-left: "" -> [w145]
          i -> [w147]
          n58 = Equal To 0?(x=w147) -> (x = 0?=w148:bool)
          n59 = Select(t="", s=w148, f=", ") -> (s? t:f=w144:string)
          n60 = Concatenate Strings(w145, w144, w143) -> (w146:string)
        }
        n61 = To Variant(anything=w135) -> (Variant=w141:variant)
      }
      frame "GEAR_toggle_results" {
        # "operation ID"
        n62 = Variant To Data(type=0 ("Row"), Variant=w166) -> (data=w163:i32)  [unwired: 1 in, 1 out]
        n63 = Unbundle By Name(w153) -> ("REPORT_GEAR_all_info.operation_statuses"=w156:T5[], "REPORT_GEAR_all_info.operations"=w161:string[][], "REPORTS_references.SQL_listbox_reference"=w167:refnum<vi>)
        n64 = property class="MCListbox (strict)"(reference=w167) -> ("ItemNames"=w164:string[][])  [unwired: 1 in, 2 out]
        n65 = Index Array(array=w164, index (row)=w163, index (col)=0 ("disabled index (col)")) -> (element=w158:string)
        n66 = Index Array(array=w161, index (col)=0 ("disabled index (col)")) -> (element=w159:string[])  [unwired: 1 in]
        n67 = Search 1D Array(1D array=w159, element=w158) -> (index of element=w154:i32)  [unwired: 1 in]
        n68 = Index Array(array=w156, index=w154) -> (element=w157:T5)
        n69 = case shown="\"OP_unexpected_show\"" w157 {
          selector: w157 -> [_ _ _ _ _ _ _ _ _ _ w179]
          tunnel: [REPORT_GEAR_statuses."OP_OK_show" ("REPORT_GEAR_statuses") REPORT_GEAR_statuses."OP_OK_hide" ("REPORT_GEAR_statuses") REPORT_GEAR_statuses."OP_NOK_show" ("REPORT_GEAR_statuses") REPORT_GEAR_statuses."OP_NOK_hide" ("REPORT_GEAR_statuses") REPORT_GEAR_statuses."OP_interrupted_show" ("REPORT_GEAR_statuses") REPORT_GEAR_statuses."OP_interrupted_hide" ("REPORT_GEAR_statuses") REPORT_GEAR_statuses."OP_in_operation_show" ("REPORT_GEAR_statuses") REPORT_GEAR_statuses."OP_in_operation_hide" ("REPORT_GEAR_statuses") REPORT_GEAR_statuses."OP_unexpected_show" ("REPORT_GEAR_statuses") REPORT_GEAR_statuses."OP_unexpected_hide" ("REPORT_GEAR_statuses") w179] -> w155
          frame "OP_OK_hide" {
          }
          frame "OP_OK_show" {
          }
          frame "OP_NOK_hide" {
          }
          frame "OP_NOK_show" {
          }
          frame "OP_interrupted_hide" {
          }
          frame "OP_interrupted_show" {
          }
          frame "OP_in_operation_hide" {
          }
          frame "OP_in_operation_show" {
          }
          frame "OP_unexpected_hide" {
          }
          frame "OP_unexpected_show" {
          }
          frame Default {
          }
        }
        n70 = Replace Array Subset(array=w156, new element=w155, index=w154) -> (w151:T5[])
        n71 = Bundle By Name(cluster=w153, "REPORT_GEAR_all_info.operation_statuses"=w151) -> (w152:T2)
      }
      frame "GEAR_show_all_results" {
        n72 = Unbundle By Name(w183) -> ("REPORT_GEAR_all_info.operation_statuses"=w181:T5[])
        n73 = for {
          tunnel: w181 -> [w186] mode=indexing
          tunnel: [w185] -> w180 mode=indexing
          n74 = case shown="\"OP_OK_hide\"" w186 {
            selector: w186 -> [_ _ _ _ _ w192]
            tunnel: [REPORT_GEAR_statuses."OP_OK_show" ("REPORT_GEAR_statuses") REPORT_GEAR_statuses."OP_NOK_show" ("REPORT_GEAR_statuses") REPORT_GEAR_statuses."OP_interrupted_show" ("REPORT_GEAR_statuses") REPORT_GEAR_statuses."OP_in_operation_show" ("REPORT_GEAR_statuses") REPORT_GEAR_statuses."OP_unexpected_show" ("REPORT_GEAR_statuses") w192] -> w185
            frame "OP_OK_hide" {
            }
            frame "OP_NOK_hide" {
            }
            frame "OP_interrupted_hide" {
            }
            frame "OP_in_operation_hide" {
            }
            frame "OP_unexpected_hide" {
            }
            frame Default {
            }
          }
        }
        n75 = Bundle By Name(cluster=w183, "REPORT_GEAR_all_info.operation_statuses"=w180) -> (w182:T2)
      }
      frame "GEAR_hide_all_results" {
        n76 = Unbundle By Name(w196) -> ("REPORT_GEAR_all_info.operation_statuses"=w194:T5[])
        n77 = for {
          tunnel: w194 -> [w198] mode=indexing
          tunnel: [w199] -> w193 mode=indexing
          n78 = case shown="\"OP_unexpected_show\"" w198 {
            selector: w198 -> [_ _ _ _ _ w205]
            tunnel: [REPORT_GEAR_statuses."OP_OK_hide" ("REPORT_GEAR_statuses") REPORT_GEAR_statuses."OP_NOK_hide" ("REPORT_GEAR_statuses") REPORT_GEAR_statuses."OP_interrupted_hide" ("REPORT_GEAR_statuses") REPORT_GEAR_statuses."OP_in_operation_hide" ("REPORT_GEAR_statuses") REPORT_GEAR_statuses."OP_unexpected_hide" ("REPORT_GEAR_statuses") w205] -> w199
            frame "OP_OK_show" {
            }
            frame "OP_NOK_show" {
            }
            frame "OP_interrupted_show" {
            }
            frame "OP_in_operation_show" {
            }
            frame "OP_unexpected_show" {
            }
            frame Default {
            }
          }
        }
        n79 = Bundle By Name(cluster=w196, "REPORT_GEAR_all_info.operation_statuses"=w193) -> (w195:T2)
      }
      frame "GEAR_display" {
        n80 = Unbundle By Name(w208) -> ("REPORTS_references.REPORT_GEAR_header_data_display"=w211:refnum<vi>, "REPORT_GEAR_all_info.REPORT_GEAR_header"=w210:T4)
        n81 = call-poly "Get Localized Phrase Compact Interface.vi"("Key"=string[] ["ID", "Time", "OP", "Status", "Operator"] ("column_names")) -> ("Translated Phrase"=w206:string[])
        n82 = call "REPORT_GEAR_listbox_set_values_and_recolor.vi"("column_names"=w206, "REPORT_all_info_in"=w208) -> ("REPORT_all_info_out"=w207:T2)  [unwired: 8 in, 1 out]
        n83 = property class="Clust (strict)"(reference=w211, "Value"=w210) -> ()  [unwired: 1 in, 2 out]
      }
      frame "GEAR_filter" {
        n84 = Variant To Data(type="", Variant=w215) -> (data=w214:string)  [unwired: 1 in, 1 out]
        n85 = call "REPORT_GEAR_listbox_filter.vi"("OP"=w214, "REPORT_all_info_in"=w216) -> ("REPORT_all_info_out"=w217:T2)  [unwired: 8 in, 1 out]
      }
      frame "GEAR_restore" {
        n86 = call "REPORT_GEAR_listbox_restore.vi"("REPORT_all_info_in"=w219) -> ()  [unwired: 10 in, 1 out]
      }
      frame "GEAR_clear" {
        n87 = Unbundle By Name(w227) -> ("REPORTS_references"=w222:T18)
        n88 = call "REPORT_GEAR_initialize_GUI.vi"("REPORTS_references_in"=w222) -> ()  [unwired: 10 in, 1 out]
        n89 = Unbundle By Name(w222) -> ("SQL_listbox_reference"=w223:refnum<vi>, "front_panel_reference"=w224:refnum<vi>)
        n90 = call "listbox_set_values_and_recolor.vi"("item_names"=string[][] [], "front_panel_reference"=w224, "column_names"=string[] [], "multicolumn_listbox_reference_in"=w223) -> ()  [unwired: 6 in, 2 out]
        n91 = Bundle By Name(cluster=w227, "REPORT_GEAR_all_info"=T3 {"serial"="", "filter_OP"="", "REPORT_GEAR_header"={"ID"="", "creation_time"="", "last_station"="", "last_status"="", "pinion_serial"="", "batch_code"=""}, "operations"=[], "operation_statuses"=[], "results"=[], "result_statuses"=[], "batches"=[], "batch_statuses"=[], "column_headers"=[], "displayed_rows"=[], "displayed_statuses"=[], "column_widths"=[]}) -> (w228:T2)
      }
      frame "GEAR_get_all_info" {
        n92 = Unbundle By Name(w232) -> ("REPORT_GEAR_all_info"=w231:T3)
        n93 = To Variant(anything=w231) -> (Variant=w230:variant)
      }
      frame "DATES_set_dates" {
        n94 = Variant To Data(type=string[] [], Variant=w243) -> (data=w241:string[])  [unwired: 1 in, 1 out]
        n95 = Index Array(array=w241, index #1=0 ("index (row)")) -> (element #1=w236:string, element #2=w235:string, element #3=w234:string, element #4=w237:string)  [unwired: 3 in]
        n96 = Bundle By Name(cluster=w239, "REPORT_DATES_all_info.date_start"=w236, "REPORT_DATES_all_info.date_end"=w235, "REPORT_DATES_all_info.time_start"=w234, "REPORT_DATES_all_info.time_end"=w237) -> (w238:T2)
      }
      frame "DATES_set_gears" {
        # "gear last status"
        n97 = Variant To Data(type=string[][] [], Variant=w254) -> (data=w248:string[][])  [unwired: 1 in, 1 out]
        n98 = Index Array(array=w248, index (col)=4 ("disabled index (col)")) -> (element=w250:string[])  [unwired: 1 in]
        n99 = for {
          tunnel: w250 -> [w259] mode=indexing
          tunnel: [w258] -> w249 mode=indexing
          tunnel: [w257] -> w245 mode=indexing
          n100 = call "REPORT_DATES_status_number_to_description_and_enum.vi"("status_nmb"=w259) -> ("status_enum"=w258:T7, "status_description"=w257:string)  [unwired: 9 in]
        }
        n101 = Replace Array Subset(array=w248, new element=w245, index (col)=4 ("disabled index (col)")) -> (w246:string[][])  [unwired: 1 in]
        n102 = Bundle By Name(cluster=w253, "REPORT_DATES_all_info.gears"=w246, "REPORT_DATES_all_info.gears_statuses"=w249) -> (w255:T2)
      }
      frame "DATES_display" {
        w261 = "ALL" ("REPORT_DATES_all_info.filter_last_OP")
        n103 = Variant To Data(type=enum32{"old_to_new", "new_to_old"}."old_to_new" ("REPORT_DATES_order_selection"), Variant=w266) -> (data=w264:enum32{"old_to_new", "new_to_old"})  [unwired: 1 in, 1 out]
        n104 = call-poly "Get Localized Phrase Compact Interface.vi"("Key"=string[] ["ID", "Time", "Gear Serial", "Last OP", "Last Status", "Pinion Serial", "Batch Code"] ("column_names")) -> ("Translated Phrase"=w260:string[])
        n105 = call "REPORT_DATES_listbox_set_values_and_recolor.vi"("column_names"=w260, "order"=w264, "REPORT_all_info_in"=w267) -> ("REPORT_all_info_out"=w263:T2)  [unwired: 7 in, 1 out]
        n106 = Bundle By Name(cluster=w263, "REPORT_DATES_all_info.filter_last_OP"=w261, "REPORT_DATES_all_info.filter_last_status"=w261) -> (w262:T2)
      }
      frame "DATES_filter" {
        n107 = Variant To Data(type=T19 {"order_selection"=enum."new_to_old", "last_OP"="", "last_status"=""}, Variant=w272) -> (data=w270:T19)  [unwired: 1 in, 1 out]
        n108 = call "REPORT_DATES_listbox_filter.vi"("REPORT_DATES_filters"=w270, "REPORT_all_info_in"=w273) -> ("REPORT_all_info_out"=w274:T2)  [unwired: 8 in, 1 out]
      }
      frame "DATES_first_page" {
        n109 = call "REPORT_DATES_change_page.vi"("REPORT_page_change"=REPORT_page_change."first", "REPORT_all_info_in"=w278) -> ("REPORT_all_info_out"=w277:T2)  [unwired: 8 in, 1 out]
      }
      frame "DATES_previous_page" {
        n110 = call "REPORT_DATES_change_page.vi"("REPORT_page_change"=REPORT_page_change."previous", "REPORT_all_info_in"=w282) -> ("REPORT_all_info_out"=w281:T2)  [unwired: 8 in, 1 out]
      }
      frame "DATES_next_page" {
        n111 = call "REPORT_DATES_change_page.vi"("REPORT_page_change"=REPORT_page_change."next", "REPORT_all_info_in"=w286) -> ("REPORT_all_info_out"=w285:T2)  [unwired: 8 in, 1 out]
      }
      frame "DATES_last_page" {
        n112 = call "REPORT_DATES_change_page.vi"("REPORT_page_change"=REPORT_page_change."last", "REPORT_all_info_in"=w290) -> ("REPORT_all_info_out"=w289:T2)  [unwired: 8 in, 1 out]
      }
      frame "DATES_restore" {
        n113 = call "REPORT_DATES_listbox_restore.vi"("REPORT_all_info_in"=w292) -> ()  [unwired: 10 in, 1 out]
      }
      frame "DATES_clear" {
        n114 = Unbundle By Name(w300) -> ("REPORTS_references"=w294:T18)
        n115 = call "REPORT_DATES_initialize_GUI.vi"("REPORTS_references_in"=w294) -> ()  [unwired: 10 in, 1 out]
        n116 = Unbundle By Name(w294) -> ("SQL_listbox_reference"=w295:refnum<vi>, "front_panel_reference"=w296:refnum<vi>)
        n117 = call "listbox_set_values_and_recolor.vi"("item_names"=string[][] [], "front_panel_reference"=w296, "column_names"=string[] [], "multicolumn_listbox_reference_in"=w295) -> ()  [unwired: 6 in, 2 out]
        n118 = Bundle By Name(cluster=w300, "REPORT_DATES_all_info"=T6 {"date_start"="", "date_end"="", "time_start"="", "time_end"="", "filter_last_OP"="", "filter_last_status"="", "gears"=[], "gears_statuses"=[], "column_headers"=[], "displayed_rows"=[], "displayed_statuses"=[], "column_widths"=[], "active_page"=0}) -> (w301:T2)
      }
      frame "DATES_get_all_info" {
        n119 = Unbundle By Name(w305) -> ("REPORT_DATES_all_info"=w304:T6)
        n120 = To Variant(anything=w304) -> (Variant=w303:variant)
      }
      frame "PBATCH_set_batch_no" {
        n121 = Variant To Data(type="", Variant=w310) -> (data=w307:string)  [unwired: 1 in, 1 out]
        n122 = Bundle By Name(cluster=w309, "REPORT_PBATCH_all_info.batch_no"=w307) -> (w311:T2)
      }
      frame "PBATCH_set_gears" {
        # "gear last status"
        n123 = Variant To Data(type=string[][] [], Variant=w322) -> (data=w316:string[][])  [unwired: 1 in, 1 out]
        n124 = Index Array(array=w316, index (col)=4 ("disabled index (col)")) -> (element=w318:string[])  [unwired: 1 in]
        n125 = for {
          tunnel: w318 -> [w327] mode=indexing
          tunnel: [w326] -> w317 mode=indexing
          tunnel: [w325] -> w313 mode=indexing
          n126 = call "REPORT_DATES_status_number_to_description_and_enum.vi"("status_nmb"=w327) -> ("status_enum"=w326:T7, "status_description"=w325:string)  [unwired: 9 in]
        }
        n127 = Replace Array Subset(array=w316, new element=w313, index (col)=4 ("disabled index (col)")) -> (w314:string[][])  [unwired: 1 in]
        n128 = Bundle By Name(cluster=w321, "REPORT_PBATCH_all_info.gears"=w314, "REPORT_PBATCH_all_info.gears_statuses"=w317) -> (w323:T2)
      }
      frame "PBATCH_display" {
        w329 = "ALL" ("REPORT_DATES_all_info.filter_last_OP")
        n129 = Variant To Data(type=enum32{"old_to_new", "new_to_old"}."old_to_new" ("REPORT_DATES_order_selection"), Variant=w334) -> (data=w332:enum32{"old_to_new", "new_to_old"})  [unwired: 1 in, 1 out]
        n130 = call-poly "Get Localized Phrase Compact Interface.vi"("Key"=string[] ["ID", "Time", "Gear Serial", "Last OP", "Last Status", "Pinion Serial", "CBatch Code", "PBatch OP"] ("column_names")) -> ("Translated Phrase"=w328:string[])
        n131 = call "REPORT_PBATCH_listbox_set_values_and_recolor.vi"("column_names"=w328, "order"=w332, "REPORT_all_info_in"=w335) -> ("REPORT_all_info_out"=w331:T2)  [unwired: 7 in, 1 out]
        n132 = Bundle By Name(cluster=w331, "REPORT_PBATCH_all_info.filter_last_OP"=w329, "REPORT_PBATCH_all_info.filter_last_status"=w329) -> (w330:T2)
      }
      frame "PBATCH_filter" {
        n133 = Variant To Data(type=T21 {"order_selection"=enum."new_to_old", "last_OP"="", "last_status"=""} ("REPORT_DATES_filters"), Variant=w342) -> (data=w338:T21)  [unwired: 1 in, 1 out]
        n134 = call "REPORT_PBATCH_listbox_filter.vi"("REPORT_PBATCH_filters"=w338, "REPORT_all_info_in"=w341) -> ("REPORT_all_info_out"=w340:T2)  [unwired: 8 in, 1 out]
      }
      frame "PBATCH_first_page" {
        n135 = call "REPORT_PBATCH_change_page.vi"("REPORT_page_change"=REPORT_page_change."first", "REPORT_all_info_in"=w346) -> ("REPORT_all_info_out"=w345:T2)  [unwired: 8 in, 1 out]
      }
      frame "PBATCH_previous_page" {
        n136 = call "REPORT_PBATCH_change_page.vi"("REPORT_page_change"=REPORT_page_change."previous", "REPORT_all_info_in"=w350) -> ("REPORT_all_info_out"=w349:T2)  [unwired: 8 in, 1 out]
      }
      frame "PBATCH_next_page" {
        n137 = call "REPORT_PBATCH_change_page.vi"("REPORT_page_change"=REPORT_page_change."next", "REPORT_all_info_in"=w354) -> ("REPORT_all_info_out"=w353:T2)  [unwired: 8 in, 1 out]
      }
      frame "PBATCH_last_page" {
        n138 = call "REPORT_PBATCH_change_page.vi"("REPORT_page_change"=REPORT_page_change."last", "REPORT_all_info_in"=w358) -> ("REPORT_all_info_out"=w357:T2)  [unwired: 8 in, 1 out]
      }
      frame "PBATCH_restore" {
        n139 = call "REPORT_PBATCH_listbox_restore.vi"("REPORT_all_info_in"=w360) -> ()  [unwired: 10 in, 1 out]
      }
      frame "PBATCH_clear" {
        n140 = Unbundle By Name(w368) -> ("REPORTS_references"=w363:T18)
        n141 = call "REPORT_PBATCH_initialize_GUI.vi"("REPORTS_references_in"=w363) -> ()  [unwired: 10 in, 1 out]
        n142 = Unbundle By Name(w363) -> ("SQL_listbox_reference"=w364:refnum<vi>, "front_panel_reference"=w365:refnum<vi>)
        n143 = call "listbox_set_values_and_recolor.vi"("item_names"=string[][] [], "front_panel_reference"=w365, "column_names"=string[] [], "multicolumn_listbox_reference_in"=w364) -> ()  [unwired: 6 in, 2 out]
        n144 = Bundle By Name(cluster=w368, "REPORT_PBATCH_all_info"=T8 {"batch_no"="", "filter_last_OP"="", "filter_last_status"="", "gears"=[], "gears_statuses"=[], "column_headers"=[], "displayed_rows"=[], "displayed_statuses"=[], "column_widths"=[], "active_page"=0}) -> (w369:T2)
      }
      frame "PBATCH_get_all_info" {
        n145 = Unbundle By Name(w373) -> ("REPORT_PBATCH_all_info"=w372:T8)
        n146 = To Variant(anything=w372) -> (Variant=w371:variant)
      }
      frame "OPRTN_set_OP" {
        n147 = Variant To Data(type="", Variant=w378) -> (data=w375:string)  [unwired: 1 in, 1 out]
        n148 = Bundle By Name(cluster=w377, "REPORT_OPRTN_all_info.OP"=w375) -> (w379:T2)
      }
      frame "OPRTN_set_dates" {
        n149 = Variant To Data(type=string[] [], Variant=w390) -> (data=w388:string[])  [unwired: 1 in, 1 out]
        n150 = Index Array(array=w388, index #1=0 ("index (row)")) -> (element #1=w383:string, element #2=w382:string, element #3=w381:string, element #4=w384:string)  [unwired: 3 in]
        n151 = Bundle By Name(cluster=w386, "REPORT_OPRTN_all_info.date_start"=w383, "REPORT_OPRTN_all_info.date_end"=w382, "REPORT_OPRTN_all_info.time_start"=w381, "REPORT_OPRTN_all_info.time_end"=w384) -> (w385:T2)
      }
      frame "OPRTN_set_gears" {
        w396 = 1 ("disabled index (col)")
        w404 = 6 ("index (col)")
        # "gear last status\nvalue"
        n152 = Variant To Data(type=string[][] [], Variant=w408) -> (data=w402:string[][])  [unwired: 1 in, 1 out]
        n153 = Index Array(array=w402, index (col)=w404) -> (element=w405:string[])  [unwired: 1 in]
        n154 = disable-structure shown="Enabled" {
          disable-tunnel: w405 -> [w412 w416]
          disable-tunnel: [w411 w415] -> w403
          frame Disabled {
            n155 = for {
              tunnel: w412 -> [w414] mode=indexing
              tunnel: [w413] -> w411 mode=indexing
              n156 = call "first_coma_to_period.vi"("string_in"=w414) -> ("string_out"=w413:string)  [unwired: 10 in]
            }
          }
          frame Enabled {
            n157 = call "REPORT_OPRTN_reformat_reals.vi"("reals_in"=w416) -> ("reals_out"=w415:string[])  [unwired: 10 in]
          }
        }
        n158 = Replace Array Subset(array=w402, new element=w403, index (col)=w404) -> (w401:string[][])  [unwired: 1 in]
        n159 = call "REPORT_OPRTN_reshape_records_for_display.vi"("records_from_SQL"=w401) -> ("records_to_display"=w398:string[][], "archivisation_description"=w393:string[][], "column_headers"=w394:string[], "number_of_static_columns"=w392:i32)  [unwired: 7 in]
        n160 = Index Array(array=w398, index (col)=w396) -> (element=w400:string[])  [unwired: 1 in]
        n161 = for {
          tunnel: w400 -> [w419] mode=indexing
          tunnel: [w418] -> w395 mode=indexing
          tunnel: [w417] -> w399 mode=indexing
          n162 = call "REPORT_DATES_status_number_to_description_and_enum.vi"("status_nmb"=w419) -> ("status_enum"=w417:T7, "status_description"=w418:string)  [unwired: 9 in]
        }
        n163 = Replace Array Subset(array=w398, new element=w395, index (col)=w396) -> (w397:string[][])  [unwired: 1 in]
        n164 = Bundle By Name(cluster=w407, "REPORT_OPRTN_all_info.no_of_static_columns"=w392, "REPORT_OPRTN_all_info.column_headers"=w394, "REPORT_OPRTN_all_info.operations"=w397, "REPORT_OPRTN_all_info.operations_statuses"=w399, "REPORT_OPRTN_all_info.archivisation_description"=w393) -> (w409:T2)
      }
      frame "OPRTN_set_hidden_columns" {
        n165 = Variant To Data(type=i32[] [] ("x+y"), Variant=w424) -> (data=w420:i32[])  [unwired: 1 in, 1 out]
        n166 = Bundle By Name(cluster=w423, "REPORT_OPRTN_all_info.hidden_columns"=w420) -> (w422:T2)
      }
      frame "OPRTN_display" {
        n167 = Variant To Data(type=enum32{"old_to_new", "new_to_old"}."old_to_new" ("REPORT_DATES_order_selection"), Variant=w432) -> (data=w430:enum32{"old_to_new", "new_to_old"})  [unwired: 1 in, 1 out]
        n168 = call "REPORT_OPRTN_listbox_set_values_and_recolor.vi"("order"=w430, "REPORT_all_info_in"=w433) -> ("REPORT_all_info_out"=w429:T2)  [unwired: 8 in, 1 out]
        n169 = Bundle By Name(cluster=w429, "REPORT_OPRTN_all_info.filter_last_status"="ALL" ("REPORT_DATES_all_info.filter_last_OP"), "REPORT_OPRTN_all_info.hidden_columns"=i32[] []) -> (w428:T2)
      }
      frame "OPRTN_filter" {
        n170 = Variant To Data(type=T22 {"order_selection"=enum."new_to_old", "last_status"=""} ("REPORT_DATES_filters"), Variant=w440) -> (data=w436:T22)  [unwired: 1 in, 1 out]
        n171 = call "REPORT_OPRTN_listbox_filter.vi"("reset_page?"=TRUE, "REPORT_OPRTN_filters"=w436, "REPORT_all_info_in"=w439) -> ("REPORT_all_info_out"=w438:T2)  [unwired: 7 in, 1 out]
      }
      frame "OPRTN_filter_no_page_reset" {
        n172 = Variant To Data(type=T22 {"order_selection"=enum."new_to_old", "last_status"=""} ("REPORT_DATES_filters"), Variant=w447) -> (data=w443:T22)  [unwired: 1 in, 1 out]
        n173 = call "REPORT_OPRTN_listbox_filter.vi"("reset_page?"=FALSE, "REPORT_OPRTN_filters"=w443, "REPORT_all_info_in"=w446) -> ("REPORT_all_info_out"=w445:T2)  [unwired: 7 in, 1 out]
      }
      frame "OPRTN_first_page" {
        n174 = call "REPORT_OPRTN_change_page.vi"("REPORT_page_change"=REPORT_page_change."first", "REPORT_all_info_in"=w451) -> ("REPORT_all_info_out"=w450:T2)  [unwired: 8 in, 1 out]
      }
      frame "OPRTN_previous_page" {
        n175 = call "REPORT_OPRTN_change_page.vi"("REPORT_page_change"=REPORT_page_change."previous", "REPORT_all_info_in"=w455) -> ("REPORT_all_info_out"=w454:T2)  [unwired: 8 in, 1 out]
      }
      frame "OPRTN_next_page" {
        n176 = call "REPORT_OPRTN_change_page.vi"("REPORT_page_change"=REPORT_page_change."next", "REPORT_all_info_in"=w459) -> ("REPORT_all_info_out"=w458:T2)  [unwired: 8 in, 1 out]
      }
      frame "OPRTN_last_page" {
        n177 = call "REPORT_OPRTN_change_page.vi"("REPORT_page_change"=REPORT_page_change."last", "REPORT_all_info_in"=w463) -> ("REPORT_all_info_out"=w462:T2)  [unwired: 8 in, 1 out]
      }
      frame "OPRTN_restore" {
        n178 = call "REPORT_OPRTN_listbox_restore.vi"("REPORT_all_info_in"=w465) -> ()  [unwired: 10 in, 1 out]
      }
      frame "OPRTN_clear" {
        n179 = Unbundle By Name(w473) -> ("REPORTS_references"=w468:T18)
        n180 = call "REPORT_OPRTN_initialize_GUI.vi"("REPORTS_references_in"=w468) -> ()  [unwired: 10 in, 1 out]
        n181 = Unbundle By Name(w468) -> ("SQL_listbox_reference"=w469:refnum<vi>, "front_panel_reference"=w470:refnum<vi>)
        n182 = call "listbox_set_values_and_recolor.vi"("item_names"=string[][] [], "front_panel_reference"=w470, "column_names"=string[] [], "multicolumn_listbox_reference_in"=w469) -> ()  [unwired: 6 in, 2 out]
        n183 = Bundle By Name(cluster=w473, "REPORT_OPRTN_all_info"=T9 {"OP"="", "date_start"="", "date_end"="", "time_start"="", "time_end"="", "filter_last_status"="", "no_of_static_columns"=0, "operations"=[], "operations_statuses"=[], "column_headers"=[], "archivisation_description"=[], "displayed_rows"=[], "displayed_statuses"=[], "column_widths"=[], "hidden_columns"=[], "active_page"=0}) -> (w474:T2)
      }
      frame "OPRTN_get_all_info" {
        n184 = Unbundle By Name(w478) -> ("REPORT_OPRTN_all_info"=w477:T9)
        n185 = To Variant(anything=w477) -> (Variant=w476:variant)
      }
      frame "CFG_set_type" {
        n186 = Variant To Data(type=REPORT_CFG_types."REFERENCE", Variant=w483) -> (data=w481:T11)  [unwired: 1 in, 1 out]
        n187 = Bundle By Name(cluster=w482, "REPORT_CFG_all_info.type"=w481) -> (w484:T2)
      }
      frame "CFG_set_dates" {
        n188 = Variant To Data(type=string[] [], Variant=w495) -> (data=w493:string[])  [unwired: 1 in, 1 out]
        n189 = Index Array(array=w493, index #1=0 ("index (row)")) -> (element #1=w488:string, element #2=w487:string, element #3=w486:string, element #4=w489:string)  [unwired: 3 in]
        n190 = Bundle By Name(cluster=w491, "REPORT_CFG_all_info.date_start"=w488, "REPORT_CFG_all_info.date_end"=w487, "REPORT_CFG_all_info.time_start"=w486, "REPORT_CFG_all_info.time_end"=w489) -> (w490:T2)
      }
      frame "CFG_set_records" {
        n191 = Unbundle By Name(w500) -> ("REPORT_CFG_all_info.type"=w499:T11)
        n192 = Variant To Data(type=string[][] [], Variant=w504) -> (data=w501:string[][])  [unwired: 1 in, 1 out]
        n193 = case shown="\"ARCHIVISATION\"" w499 {
          tunnel: [string[] ["Archivisation Time", "Creation Time", "Reference Name", "OP", "Description", "Value", "Unit", "Tag Type", "Tag Address", "Created By", "Deleted By"] string[] ["Archivisation Time", "Creation Time", "Reference Name", "OP", "Description", "Unit", "Tag Type", "Tag Address", "Created By", "Deleted By"] string[] ["Archivisation Time", "Creation Time", "User Name", "User No", "Description", "10", "20", "30", "40", "50", "60", "70", "80", "90", "100", "110", "120", "130", "140", "150", "160", "165", "Trace App", "Barcode Hash", "Created By", "Deleted By"]] -> w498
          frame "REFERENCE" {
          }
          frame "ARCHIVISATION" {
          }
          frame "USERS" {
          }
        }
        n194 = call-poly "Get Localized Phrase Compact Interface.vi"("Key"=w498) -> ("Translated Phrase"=w497:string[])
        n195 = Bundle By Name(cluster=w500, "REPORT_CFG_all_info.column_headers"=w497, "REPORT_CFG_all_info.records"=w501) -> (w503:T2)
      }
      frame "CFG_display" {
        n196 = Variant To Data(type=enum32{"old_to_new", "new_to_old"}."old_to_new" ("REPORT_DATES_order_selection"), Variant=w514) -> (data=w512:enum32{"old_to_new", "new_to_old"})  [unwired: 1 in, 1 out]
        n197 = call "REPORT_CFG_listbox_set_values_and_recolor.vi"("order"=w512, "REPORT_all_info_in"=w515) -> ("REPORT_all_info_out"=w511:T2)  [unwired: 8 in, 1 out]
        n198 = Bundle By Name(cluster=w511, "REPORT_CFG_all_info.filter_OP"="ALL" ("REPORT_DATES_all_info.filter_last_OP")) -> (w510:T2)
      }
      frame "CFG_filter" {
        n199 = Variant To Data(type=T23 {"order_selection"=enum."new_to_old", "OP"=""} ("REPORT_DATES_filters"), Variant=w521) -> (data=w518:T23)  [unwired: 1 in, 1 out]
        n200 = call "REPORT_CFG_listbox_filter.vi"("REPORT_CFG_filters"=w518, "REPORT_all_info_in"=w520) -> ("REPORT_all_info_out"=w519:T2)  [unwired: 8 in, 1 out]
      }
      frame "CFG_first_page" {
        n201 = call "REPORT_CFG_change_page.vi"("REPORT_page_change"=REPORT_page_change."first", "REPORT_all_info_in"=w525) -> ("REPORT_all_info_out"=w524:T2)  [unwired: 8 in, 1 out]
      }
      frame "CFG_previous_page" {
        n202 = call "REPORT_CFG_change_page.vi"("REPORT_page_change"=REPORT_page_change."previous", "REPORT_all_info_in"=w529) -> ("REPORT_all_info_out"=w528:T2)  [unwired: 8 in, 1 out]
      }
      frame "CFG_next_page" {
        n203 = call "REPORT_CFG_change_page.vi"("REPORT_page_change"=REPORT_page_change."next", "REPORT_all_info_in"=w533) -> ("REPORT_all_info_out"=w532:T2)  [unwired: 8 in, 1 out]
      }
      frame "CFG_last_page" {
        n204 = call "REPORT_CFG_change_page.vi"("REPORT_page_change"=REPORT_page_change."last", "REPORT_all_info_in"=w537) -> ("REPORT_all_info_out"=w536:T2)  [unwired: 8 in, 1 out]
      }
      frame "CFG_restore" {
        n205 = call "REPORT_CFG_listbox_restore.vi"("REPORT_all_info_in"=w539) -> ()  [unwired: 10 in, 1 out]
      }
      frame "CFG_clear" {
        n206 = Unbundle By Name(w547) -> ("REPORTS_references"=w542:T18)
        n207 = call "REPORT_CFG_initialize_GUI.vi"("REPORTS_references_in"=w542) -> ()  [unwired: 10 in, 1 out]
        n208 = Unbundle By Name(w542) -> ("SQL_listbox_reference"=w543:refnum<vi>, "front_panel_reference"=w544:refnum<vi>)
        n209 = call "listbox_set_values_and_recolor.vi"("item_names"=string[][] [], "front_panel_reference"=w544, "column_names"=string[] [], "multicolumn_listbox_reference_in"=w543) -> ()  [unwired: 6 in, 2 out]
        n210 = Bundle By Name(cluster=w547, "REPORT_CFG_all_info"=T10 {"type"=enum."REFERENCE", "date_start"="", "date_end"="", "time_start"="", "time_end"="", "filter_OP"="", "records"=[], "column_headers"=[], "displayed_rows"=[], "column_widths"=[], "active_page"=0}) -> (w548:T2)
      }
      frame "CFG_get_all_info" {
        n211 = Unbundle By Name(w552) -> ("REPORT_CFG_all_info"=w551:T10)
        n212 = To Variant(anything=w551) -> (Variant=w550:variant)
      }
      frame "AUDIT_set_dates" {
        n213 = Variant To Data(type=string[] [], Variant=w563) -> (data=w561:string[])  [unwired: 1 in, 1 out]
        n214 = Index Array(array=w561, index #1=0 ("index (row)")) -> (element #1=w556:string, element #2=w555:string, element #3=w554:string, element #4=w557:string)  [unwired: 3 in]
        n215 = Bundle By Name(cluster=w559, "REPORT_AUDIT_all_info.date_start"=w556, "REPORT_AUDIT_all_info.date_end"=w555, "REPORT_AUDIT_all_info.time_start"=w554, "REPORT_AUDIT_all_info.time_end"=w557) -> (w558:T2)
      }
      frame "AUDIT_set_records" {
        # "audit status"
        n216 = Variant To Data(type=string[][] [], Variant=w574) -> (data=w568:string[][])  [unwired: 1 in, 1 out]
        n217 = Index Array(array=w568, index (col)=2 ("disabled index (col)")) -> (element=w570:string[])  [unwired: 1 in]
        n218 = for {
          tunnel: w570 -> [w579] mode=indexing
          tunnel: [w578] -> w569 mode=indexing
          tunnel: [w577] -> w565 mode=indexing
          n219 = call "REPORT_DATES_status_number_to_description_and_enum.vi"("status_nmb"=w579) -> ("status_enum"=w578:T7, "status_description"=w577:string)  [unwired: 9 in]
        }
        n220 = Replace Array Subset(array=w568, new element=w565, index (col)=2 ("disabled index (col)")) -> (w566:string[][])  [unwired: 1 in]
        n221 = Bundle By Name(cluster=w573, "REPORT_AUDIT_all_info.records"=w566, "REPORT_AUDIT_all_info.record_statuses"=w569) -> (w575:T2)
      }
      frame "AUDIT_display" {
        w581 = "ALL" ("REPORT_DATES_all_info.filter_last_OP")
        n222 = Variant To Data(type=enum32{"old_to_new", "new_to_old"}."old_to_new" ("REPORT_DATES_order_selection"), Variant=w586) -> (data=w584:enum32{"old_to_new", "new_to_old"})  [unwired: 1 in, 1 out]
        n223 = call-poly "Get Localized Phrase Compact Interface.vi"("Key"=string[] ["Audit Time", "OP", "Audit Result", "User"] ("column_names")) -> ("Translated Phrase"=w580:string[])
        n224 = call "REPORT_AUDIT_listbox_set_values_and_recolor.vi"("column_names"=w580, "order"=w584, "REPORT_all_info_in"=w587) -> ("REPORT_all_info_out"=w583:T2)  [unwired: 7 in, 1 out]
        n225 = Bundle By Name(cluster=w583, "REPORT_AUDIT_all_info.filter_OP"=w581, "REPORT_AUDIT_all_info.filter_status"=w581) -> (w582:T2)
      }
      frame "AUDIT_filter" {
        n226 = Variant To Data(type=T24 {"order_selection"=enum."new_to_old", "OP_filter"="", "status_filter"=""}, Variant=w592) -> (data=w591:T24)  [unwired: 1 in, 1 out]
        n227 = call "REPORT_AUDIT_listbox_filter.vi"("REPORT_AUDIT_filters"=w591, "REPORT_all_info_in"=w593) -> ("REPORT_all_info_out"=w594:T2)  [unwired: 8 in, 1 out]
      }
      frame "AUDIT_first_page" {
        n228 = call "REPORT_AUDIT_change_page.vi"("REPORT_page_change"=REPORT_page_change."first", "REPORT_all_info_in"=w598) -> ("REPORT_all_info_out"=w597:T2)  [unwired: 8 in, 1 out]
      }
      frame "AUDIT_previous_page" {
        n229 = call "REPORT_AUDIT_change_page.vi"("REPORT_page_change"=REPORT_page_change."previous", "REPORT_all_info_in"=w602) -> ("REPORT_all_info_out"=w601:T2)  [unwired: 8 in, 1 out]
      }
      frame "AUDIT_next_page" {
        n230 = call "REPORT_AUDIT_change_page.vi"("REPORT_page_change"=REPORT_page_change."next", "REPORT_all_info_in"=w606) -> ("REPORT_all_info_out"=w605:T2)  [unwired: 8 in, 1 out]
      }
      frame "AUDIT_last_page" {
        n231 = call "REPORT_AUDIT_change_page.vi"("REPORT_page_change"=REPORT_page_change."last", "REPORT_all_info_in"=w610) -> ("REPORT_all_info_out"=w609:T2)  [unwired: 8 in, 1 out]
      }
      frame "AUDIT_restore" {
        n232 = call "REPORT_AUDIT_listbox_restore.vi"("REPORT_all_info_in"=w612) -> ()  [unwired: 10 in, 1 out]
      }
      frame "AUDIT_clear" {
        n233 = Unbundle By Name(w620) -> ("REPORTS_references"=w615:T18)
        n234 = call "REPORT_AUDIT_initialize_GUI.vi"("REPORTS_references_in"=w615) -> ()  [unwired: 10 in, 1 out]
        n235 = Unbundle By Name(w615) -> ("SQL_listbox_reference"=w616:refnum<vi>, "front_panel_reference"=w617:refnum<vi>)
        n236 = call "listbox_set_values_and_recolor.vi"("item_names"=string[][] [], "front_panel_reference"=w617, "column_names"=string[] [], "multicolumn_listbox_reference_in"=w616) -> ()  [unwired: 6 in, 2 out]
        n237 = Bundle By Name(cluster=w620, "REPORT_AUDIT_all_info"=T12 {"date_start"="", "date_end"="", "time_start"="", "time_end"="", "filter_OP"="", "filter_status"="", "records"=[], "record_statuses"=[], "column_headers"=[], "displayed_rows"=[], "displayed_statuses"=[], "column_widths"=[], "active_page"=0}) -> (w621:T2)
      }
      frame "AUDIT_get_all_info" {
        n238 = Unbundle By Name(w625) -> ("REPORT_AUDIT_all_info"=w624:T12)
        n239 = To Variant(anything=w624) -> (Variant=w623:variant)
      }
      frame "OKNOK_set_dates" {
        n240 = Variant To Data(type=string[] [], Variant=w636) -> (data=w634:string[])  [unwired: 1 in, 1 out]
        n241 = Index Array(array=w634, index #1=0 ("index (row)")) -> (element #1=w629:string, element #2=w628:string, element #3=w627:string, element #4=w630:string)  [unwired: 3 in]
        n242 = Bundle By Name(cluster=w632, "REPORT_OKNOK_all_info.date_start"=w629, "REPORT_OKNOK_all_info.date_end"=w628, "REPORT_OKNOK_all_info.time_start"=w627, "REPORT_OKNOK_all_info.time_end"=w630) -> (w631:T2)
      }
      frame "OKNOK_set_records" {
        n243 = Variant To Data(type=string[][] [], Variant=w641) -> (data=w638:string[][])  [unwired: 1 in, 1 out]
        n244 = Bundle By Name(cluster=w640, "REPORT_OKNOK_all_info.records"=w638) -> (w642:T2)
      }
      frame "OKNOK_display" {
        n245 = call-poly "Get Localized Phrase Compact Interface.vi"("Key"=string[] ["OP", "OK Count", "NOK Count"] ("column_names")) -> ("Translated Phrase"=w644:string[])
        n246 = call "REPORT_OKNOK_listbox_set_values_and_recolor.vi"("column_names"=w644, "REPORT_all_info_in"=w646) -> ("REPORT_all_info_out"=w645:T2)  [unwired: 8 in, 1 out]
      }
      frame "OKNOK_restore" {
        n247 = call "REPORT_OKNOK_listbox_restore.vi"("REPORT_all_info_in"=w649) -> ()  [unwired: 10 in, 1 out]
      }
      frame "OKNOK_clear" {
        n248 = Unbundle By Name(w657) -> ("REPORTS_references"=w652:T18)
        n249 = call "REPORT_OKNOK_initialize_GUI.vi"("REPORTS_references_in"=w652) -> ()  [unwired: 10 in, 1 out]
        n250 = Unbundle By Name(w652) -> ("SQL_listbox_reference"=w653:refnum<vi>, "front_panel_reference"=w654:refnum<vi>)
        n251 = call "listbox_set_values_and_recolor.vi"("item_names"=string[][] [], "front_panel_reference"=w654, "column_names"=string[] [], "multicolumn_listbox_reference_in"=w653) -> ()  [unwired: 6 in, 2 out]
        n252 = Bundle By Name(cluster=w657, "REPORT_OKNOK_all_info"=T13 {"date_start"="", "date_end"="", "time_start"="", "time_end"="", "records"=[], "column_headers"=[], "column_widths"=[]}) -> (w658:T2)
      }
      frame "OKNOK_get_all_info" {
        n253 = Unbundle By Name(w662) -> ("REPORT_OKNOK_all_info"=w661:T13)
        n254 = To Variant(anything=w661) -> (Variant=w660:variant)
      }
      frame "REWORKS_set_dates" {
        n255 = Variant To Data(type=string[] [], Variant=w673) -> (data=w671:string[])  [unwired: 1 in, 1 out]
        n256 = Index Array(array=w671, index #1=0 ("index (row)")) -> (element #1=w666:string, element #2=w665:string, element #3=w664:string, element #4=w667:string)  [unwired: 3 in]
        n257 = Bundle By Name(cluster=w669, "REPORT_REWORKS_all_info.date_start"=w666, "REPORT_REWORKS_all_info.date_end"=w665, "REPORT_REWORKS_all_info.time_start"=w664, "REPORT_REWORKS_all_info.time_end"=w667) -> (w668:T2)
      }
      frame "REWORKS_set_from_to" {
        w679 = T25[] [] items=["10"=10, "20"=20, "30"=30, "40"=40, "50"=50, "60"=60, "70"=70, "80"=80, "90"=90, "100"=100, "110"=110, "120"=120, "130"=130, "140"=140, "150"=150, "160"=160, "165"=165] ("appended array")
        n258 = Variant To Data(type=w679, Variant=w681) -> (data=w678:T25[])  [unwired: 1 in, 1 out]
        n259 = Number To Decimal String(number=w678) -> (decimal integer string=w677:string[])  [unwired: 1 in]
        n260 = Index Array(array=w677) -> (element #1=w676:string, element #2=w675:string)  [unwired: 2 in]
        n261 = Bundle By Name(cluster=w680, "REPORT_REWORKS_all_info.from_OP"=w676, "REPORT_REWORKS_all_info.to_OP"=w675) -> (w682:T2)
      }
      frame "REWORKS_set_records" {
        # "gear last status"
        n262 = Variant To Data(type=string[][] [], Variant=w693) -> (data=w687:string[][])  [unwired: 1 in, 1 out]
        n263 = Index Array(array=w687, index (col)=3 ("disabled index (col)")) -> (element=w689:string[])  [unwired: 1 in]
        n264 = for {
          tunnel: w689 -> [w698] mode=indexing
          tunnel: [w697] -> w688 mode=indexing
          tunnel: [w696] -> w684 mode=indexing
          n265 = call "REPORT_DATES_status_number_to_description_and_enum.vi"("status_nmb"=w698) -> ("status_enum"=w697:T7, "status_description"=w696:string)  [unwired: 9 in]
        }
        n266 = Replace Array Subset(array=w687, new element=w684, index (col)=3 ("disabled index (col)")) -> (w685:string[][])  [unwired: 1 in]
        n267 = Bundle By Name(cluster=w692, "REPORT_REWORKS_all_info.records"=w685, "REPORT_REWORKS_all_info.record_statuses"=w688) -> (w694:T2)
      }
      frame "REWORKS_display" {
        n268 = Variant To Data(type=enum32{"old_to_new", "new_to_old"}."old_to_new" ("REPORT_DATES_order_selection"), Variant=w703) -> (data=w701:enum32{"old_to_new", "new_to_old"})  [unwired: 1 in, 1 out]
        n269 = call-poly "Get Localized Phrase Compact Interface.vi"("Key"=string[] ["Gear Serial", "Time", "Last OP", "Last Status", "Pinion Serial", "Batch Code"] ("column_names")) -> ("Translated Phrase"=w699:string[])
        n270 = call "REPORT_REWORKS_listbox_set_values_and_recolor.vi"("column_names"=w699, "order"=w701, "REPORT_all_info_in"=w704) -> ("REPORT_all_info_out"=w700:T2)  [unwired: 7 in, 1 out]
      }
      frame "REWORKS_filter" {
        n271 = Variant To Data(type=enum32{"old_to_new", "new_to_old"}."old_to_new" ("REPORT_DATES_order_selection"), Variant=w709) -> (data=w707:enum32{"old_to_new", "new_to_old"})  [unwired: 1 in, 1 out]
        n272 = call "REPORT_REWORKS_listbox_filter.vi"("order_selection"=w707, "REPORT_all_info_in"=w710) -> ("REPORT_all_info_out"=w711:T2)  [unwired: 8 in, 1 out]
      }
      frame "REWORKS_first_page" {
        n273 = call "REPORT_REWORKS_change_page.vi"("REPORT_page_change"=REPORT_page_change."first", "REPORT_all_info_in"=w715) -> ("REPORT_all_info_out"=w714:T2)  [unwired: 8 in, 1 out]
      }
      frame "REWORKS_previous_page" {
        n274 = call "REPORT_REWORKS_change_page.vi"("REPORT_page_change"=REPORT_page_change."previous", "REPORT_all_info_in"=w719) -> ("REPORT_all_info_out"=w718:T2)  [unwired: 8 in, 1 out]
      }
      frame "REWORKS_next_page" {
        n275 = call "REPORT_REWORKS_change_page.vi"("REPORT_page_change"=REPORT_page_change."next", "REPORT_all_info_in"=w723) -> ("REPORT_all_info_out"=w722:T2)  [unwired: 8 in, 1 out]
      }
      frame "REWORKS_last_page" {
        n276 = call "REPORT_REWORKS_change_page.vi"("REPORT_page_change"=REPORT_page_change."last", "REPORT_all_info_in"=w727) -> ("REPORT_all_info_out"=w726:T2)  [unwired: 8 in, 1 out]
      }
      frame "REWORKS_restore" {
        n277 = call "REPORT_REWORKS_listbox_restore.vi"("REPORT_all_info_in"=w729) -> ()  [unwired: 10 in, 1 out]
      }
      frame "REWORKS_clear" {
        n278 = Unbundle By Name(w737) -> ("REPORTS_references"=w732:T18)
        n279 = call "REPORT_REWORKS_initialize_GUI.vi"("REPORTS_references_in"=w732) -> ()  [unwired: 10 in, 1 out]
        n280 = Unbundle By Name(w732) -> ("SQL_listbox_reference"=w733:refnum<vi>, "front_panel_reference"=w734:refnum<vi>)
        n281 = call "listbox_set_values_and_recolor.vi"("item_names"=string[][] [], "front_panel_reference"=w734, "column_names"=string[] [], "multicolumn_listbox_reference_in"=w733) -> ()  [unwired: 6 in, 2 out]
        n282 = Bundle By Name(cluster=w737, "REPORT_REWORKS_all_info"=T14 {"date_start"="", "date_end"="", "time_start"="", "time_end"="", "from_OP"="", "to_OP"="", "records"=[], "record_statuses"=[], "column_headers"=[], "displayed_rows"=[], "displayed_statuses"=[], "column_widths"=[], "active_page"=0}) -> (w738:T2)
      }
      frame "REWORKS_get_all_info" {
        n283 = Unbundle By Name(w742) -> ("REPORT_REWORKS_all_info"=w741:T14)
        n284 = To Variant(anything=w741) -> (Variant=w740:variant)
      }
      frame "PACE_set_dates" {
        n285 = Variant To Data(type=string[] [], Variant=w753) -> (data=w751:string[])  [unwired: 1 in, 1 out]
        n286 = Index Array(array=w751, index #1=0 ("index (row)")) -> (element #1=w746:string, element #2=w745:string, element #3=w744:string, element #4=w747:string)  [unwired: 3 in]
        n287 = Bundle By Name(cluster=w749, "REPORT_PACE_all_info.date_start"=w746, "REPORT_PACE_all_info.date_end"=w745, "REPORT_PACE_all_info.time_start"=w744, "REPORT_PACE_all_info.time_end"=w747) -> (w748:T2)
      }
      frame "PACE_set_limits" {
        n288 = Variant To Data(type=u16[] [] ("low_limit_high_limit"), Variant=w760) -> (data=w755:u16[])  [unwired: 1 in, 1 out]
        n289 = Index Array(array=w755) -> (element #1=w758:u16, element #2=w757:u16)  [unwired: 2 in]
        n290 = Bundle By Name(cluster=w759, "REPORT_PACE_all_info.low_limit"=w758, "REPORT_PACE_all_info.high_limit"=w757) -> (w761:T2)
      }
      frame "PACE_set_records" {
        n291 = Variant To Data(type=string[][] [], Variant=w766) -> (data=w763:string[][])  [unwired: 1 in, 1 out]
        n292 = Bundle By Name(cluster=w765, "REPORT_PACE_all_info.records"=w763) -> (w767:T2)
      }
      frame "PACE_display" {
        n293 = call-poly "Get Localized Phrase Compact Interface.vi"("Key"=string[] ["OP", "Count", "Operator MIN", "MIN", "AVG", "MAX", "Operator MAX"] ("column_names")) -> ("Translated Phrase"=w769:string[])
        n294 = call "REPORT_PACE_listbox_set_values_and_recolor.vi"("column_names"=w769, "REPORT_all_info_in"=w771) -> ("REPORT_all_info_out"=w770:T2)  [unwired: 8 in, 1 out]
      }
      frame "PACE_restore" {
        n295 = call "REPORT_PACE_listbox_restore.vi"("REPORT_all_info_in"=w774) -> ()  [unwired: 10 in, 1 out]
      }
      frame "PACE_clear" {
        n296 = Unbundle By Name(w782) -> ("REPORTS_references"=w777:T18)
        n297 = call "REPORT_PACE_initialize_GUI.vi"("REPORTS_references_in"=w777) -> ()  [unwired: 10 in, 1 out]
        n298 = Unbundle By Name(w777) -> ("SQL_listbox_reference"=w778:refnum<vi>, "front_panel_reference"=w779:refnum<vi>)
        n299 = call "listbox_set_values_and_recolor.vi"("item_names"=string[][] [], "front_panel_reference"=w779, "column_names"=string[] [], "multicolumn_listbox_reference_in"=w778) -> ()  [unwired: 6 in, 2 out]
        n300 = Bundle By Name(cluster=w782, "REPORT_PACE_all_info"=T15 {"date_start"="", "date_end"="", "time_start"="", "time_end"="", "low_limit"=0, "high_limit"=0, "records"=[], "column_headers"=[], "column_widths"=[]}) -> (w783:T2)
      }
      frame "PACE_get_all_info" {
        n301 = Unbundle By Name(w787) -> ("REPORT_PACE_all_info"=w786:T15)
        n302 = To Variant(anything=w786) -> (Variant=w785:variant)
      }
      frame "CBATCH_set_code" {
        n303 = Variant To Data(type="", Variant=w793) -> (data=w789:string)  [unwired: 1 in, 1 out]
        n304 = Bundle By Name(cluster=w792, "REPORT_CBATCH_all_info.batch_code"=w789) -> (w791:T2)
      }
      frame "CBATCH_set_records" {
        # "gear last status"
        n305 = Variant To Data(type=string[][] [], Variant=w804) -> (data=w798:string[][])  [unwired: 1 in, 1 out]
        n306 = Index Array(array=w798, index (col)=3 ("disabled index (col)")) -> (element=w800:string[])  [unwired: 1 in]
        n307 = for {
          tunnel: w800 -> [w809] mode=indexing
          tunnel: [w808] -> w799 mode=indexing
          tunnel: [w807] -> w795 mode=indexing
          n308 = call "REPORT_DATES_status_number_to_description_and_enum.vi"("status_nmb"=w809) -> ("status_enum"=w808:T7, "status_description"=w807:string)  [unwired: 9 in]
        }
        n309 = Replace Array Subset(array=w798, new element=w795, index (col)=3 ("disabled index (col)")) -> (w796:string[][])  [unwired: 1 in]
        n310 = Bundle By Name(cluster=w803, "REPORT_CBATCH_all_info.records"=w796, "REPORT_CBATCH_all_info.record_statuses"=w799) -> (w805:T2)
      }
      frame "CBATCH_display" {
        n311 = Variant To Data(type=enum32{"old_to_new", "new_to_old"}."old_to_new" ("REPORT_CBATCH_order_selection"), Variant=w814) -> (data=w813:enum32{"old_to_new", "new_to_old"})  [unwired: 1 in, 1 out]
        n312 = call-poly "Get Localized Phrase Compact Interface.vi"("Key"=string[] ["Gear Serial", "Time", "Last OP", "Last Status", "Pinion Serial"] ("column_names")) -> ("Translated Phrase"=w810:string[])
        n313 = call "REPORT_CBATCH_listbox_set_values_and_recolor.vi"("column_names"=w810, "order"=w813, "REPORT_all_info_in"=w815) -> ("REPORT_all_info_out"=w812:T2)  [unwired: 7 in, 1 out]
      }
      frame "CBATCH_filter" {
        n314 = Variant To Data(type=enum32{"old_to_new", "new_to_old"}."old_to_new" ("REPORT_DATES_order_selection"), Variant=w820) -> (data=w818:enum32{"old_to_new", "new_to_old"})  [unwired: 1 in, 1 out]
        n315 = call "REPORT_CBATCH_listbox_filter.vi"("order_selection"=w818, "REPORT_all_info_in"=w821) -> ("REPORT_all_info_out"=w822:T2)  [unwired: 8 in, 1 out]
      }
      frame "CBATCH_first_page" {
        n316 = call "REPORT_CBATCH_change_page.vi"("REPORT_page_change"=REPORT_page_change."first", "REPORT_all_info_in"=w826) -> ("REPORT_all_info_out"=w825:T2)  [unwired: 8 in, 1 out]
      }
      frame "CBATCH_previous_page" {
        n317 = call "REPORT_CBATCH_change_page.vi"("REPORT_page_change"=REPORT_page_change."previous", "REPORT_all_info_in"=w830) -> ("REPORT_all_info_out"=w829:T2)  [unwired: 8 in, 1 out]
      }
      frame "CBATCH_next_page" {
        n318 = call "REPORT_CBATCH_change_page.vi"("REPORT_page_change"=REPORT_page_change."next", "REPORT_all_info_in"=w834) -> ("REPORT_all_info_out"=w833:T2)  [unwired: 8 in, 1 out]
      }
      frame "CBATCH_last_page" {
        n319 = call "REPORT_CBATCH_change_page.vi"("REPORT_page_change"=REPORT_page_change."last", "REPORT_all_info_in"=w838) -> ("REPORT_all_info_out"=w837:T2)  [unwired: 8 in, 1 out]
      }
      frame "CBATCH_restore" {
        n320 = call "REPORT_CBATCH_listbox_restore.vi"("REPORT_all_info_in"=w840) -> ()  [unwired: 10 in, 1 out]
      }
      frame "CBATCH_clear" {
        n321 = Unbundle By Name(w848) -> ("REPORTS_references"=w843:T18)
        n322 = call "REPORT_CBATCH_initialize_GUI.vi"("REPORTS_references_in"=w843) -> ()  [unwired: 10 in, 1 out]
        n323 = Unbundle By Name(w843) -> ("SQL_listbox_reference"=w844:refnum<vi>, "front_panel_reference"=w845:refnum<vi>)
        n324 = call "listbox_set_values_and_recolor.vi"("item_names"=string[][] [], "front_panel_reference"=w845, "column_names"=string[] [], "multicolumn_listbox_reference_in"=w844) -> ()  [unwired: 6 in, 2 out]
        n325 = Bundle By Name(cluster=w848, "REPORT_CBATCH_all_info"=T16 {"batch_code"="", "records"=[], "record_statuses"=[], "column_headers"=[], "displayed_rows"=[], "displayed_statuses"=[], "column_widths"=[], "active_page"=0}) -> (w849:T2)
      }
      frame "CBATCH_get_all_info" {
        n326 = Unbundle By Name(w853) -> ("REPORT_CBATCH_all_info"=w852:T16)
        n327 = To Variant(anything=w852) -> (Variant=w851:variant)
      }
      frame "CMPNT_set_serial" {
        n328 = Variant To Data(type="", Variant=w859) -> (data=w855:string)  [unwired: 1 in, 1 out]
        n329 = Bundle By Name(cluster=w858, "REPORT_CMPNT_all_info.gear_serial"=w855) -> (w857:T2)
      }
      frame "CMPNT_set_records" {
        n330 = Variant To Data(type=string[][] [], Variant=w864) -> (data=w861:string[][])  [unwired: 1 in, 1 out]
        n331 = Bundle By Name(cluster=w863, "REPORT_CMPNT_all_info.records"=w861) -> (w865:T2)
      }
      frame "CMPNT_display" {
        n332 = call-poly "Get Localized Phrase Compact Interface.vi"("Key"=string[] ["Time", "OP", "Description", "Part Number", "Batch Number"] ("column_names")) -> ("Translated Phrase"=w867:string[])
        n333 = call "REPORT_CMPNT_listbox_set_values_and_recolor.vi"("column_names"=w867, "REPORT_all_info_in"=w869) -> ("REPORT_all_info_out"=w868:T2)  [unwired: 8 in, 1 out]
      }
      frame "CMPNT_first_page" {
        n334 = call "REPORT_CMPNT_change_page.vi"("REPORT_page_change"=REPORT_page_change."first", "REPORT_all_info_in"=w874) -> ("REPORT_all_info_out"=w873:T2)  [unwired: 8 in, 1 out]
      }
      frame "CMPNT_previous_page" {
        n335 = call "REPORT_CMPNT_change_page.vi"("REPORT_page_change"=REPORT_page_change."previous", "REPORT_all_info_in"=w878) -> ("REPORT_all_info_out"=w877:T2)  [unwired: 8 in, 1 out]
      }
      frame "CMPNT_next_page" {
        n336 = call "REPORT_CMPNT_change_page.vi"("REPORT_page_change"=REPORT_page_change."next", "REPORT_all_info_in"=w882) -> ("REPORT_all_info_out"=w881:T2)  [unwired: 8 in, 1 out]
      }
      frame "CMPNT_last_page" {
        n337 = call "REPORT_CMPNT_change_page.vi"("REPORT_page_change"=REPORT_page_change."last", "REPORT_all_info_in"=w886) -> ("REPORT_all_info_out"=w885:T2)  [unwired: 8 in, 1 out]
      }
      frame "CMPNT_restore" {
        n338 = call "REPORT_CMPNT_listbox_restore.vi"("REPORT_all_info_in"=w888) -> ()  [unwired: 10 in, 1 out]
      }
      frame "CMPNT_clear" {
        n339 = Unbundle By Name(w896) -> ("REPORTS_references"=w891:T18)
        n340 = call "REPORT_CMPNT_initialize_GUI.vi"("REPORTS_references_in"=w891) -> ()  [unwired: 10 in, 1 out]
        n341 = Unbundle By Name(w891) -> ("SQL_listbox_reference"=w892:refnum<vi>, "front_panel_reference"=w893:refnum<vi>)
        n342 = call "listbox_set_values_and_recolor.vi"("item_names"=string[][] [], "front_panel_reference"=w893, "column_names"=string[] [], "multicolumn_listbox_reference_in"=w892) -> ()  [unwired: 6 in, 2 out]
        n343 = Bundle By Name(cluster=w896, "REPORT_CMPNT_all_info"=T17 {"gear_serial"="", "records"=[], "column_headers"=[], "displayed_rows"=[], "column_widths"=[], "active_page"=0}) -> (w897:T2)
      }
      frame "CMPNT_get_all_info" {
        n344 = Unbundle By Name(w901) -> ("REPORT_CMPNT_all_info"=w900:T17)
        n345 = To Variant(anything=w900) -> (Variant=w899:variant)
      }
      frame "clear" {
        n346 = Unbundle By Name(w908) -> ("REPORTS_references"=w904:T18, "REPORTS_references.SQL_listbox_reference"=w907:refnum<vi>, "REPORTS_references.front_panel_reference"=w906:refnum<vi>)
        n347 = call "listbox_set_values_and_recolor.vi"("item_names"=string[][] [], "front_panel_reference"=w906, "column_names"=string[] [], "multicolumn_listbox_reference_in"=w907) -> ()  [unwired: 6 in, 2 out]
        n348 = Bundle By Name(cluster=T2 {"REPORT_GEAR_all_info"={"serial"="", "filter_OP"="", "REPORT_GEAR_header"={"ID"="", "creation_time"="", "last_station"="", "last_status"="", "pinion_serial"="", "batch_code"=""}, "operations"=[], "operation_statuses"=[], "results"=[], "result_statuses"=[], "batches"=[], "batch_statuses"=[], "column_headers"=[], "displayed_rows"=[], "displayed_statuses"=[], "column_widths"=[]}, "REPORT_DATES_all_info"={"date_start"="", "date_end"="", "time_start"="", "time_end"="", "filter_last_OP"="", "filter_last_status"="", "gears"=[], "gears_statuses"=[], "column_headers"=[], "displayed_rows"=[], "displayed_statuses"=[], "column_widths"=[], "active_page"=0}, "REPORT_PBATCH_all_info"={"batch_no"="", "filter_last_OP"="", "filter_last_status"="", "gears"=[], "gears_statuses"=[], "column_headers"=[], "displayed_rows"=[], "displayed_statuses"=[], "column_widths"=[], "active_page"=0}, "REPORT_OPRTN_all_info"={"OP"="", "date_start"="", "date_end"="", "time_start"="", "time_end"="", "filter_last_status"="", "no_of_static_columns"=0, "operations"=[], "operations_statuses"=[], "column_headers"=[], "archivisation_description"=[], "displayed_rows"=[], "displayed_statuses"=[], "column_widths"=[], "hidden_columns"=[], "active_page"=0}, "REPORT_CFG_all_info"={"type"=enum."REFERENCE", "date_start"="", "date_end"="", "time_start"="", "time_end"="", "filter_OP"="", "records"=[], "column_headers"=[], "displayed_rows"=[], "column_widths"=[], "active_page"=0}, "REPORT_AUDIT_all_info"={"date_start"="", "date_end"="", "time_start"="", "time_end"="", "filter_OP"="", "filter_status"="", "records"=[], "record_statuses"=[], "column_headers"=[], "displayed_rows"=[], "displayed_statuses"=[], "column_widths"=[], "active_page"=0}, "REPORT_OKNOK_all_info"={"date_start"="", "date_end"="", "time_start"="", "time_end"="", "records"=[], "column_headers"=[], "column_widths"=[]}, "REPORT_REWORKS_all_info"={"date_start"="", "date_end"="", "time_start"="", "time_end"="", "from_OP"="", "to_OP"="", "records"=[], "record_statuses"=[], "column_headers"=[], "displayed_rows"=[], "displayed_statuses"=[], "column_widths"=[], "active_page"=0}, "REPORT_PACE_all_info"={"date_start"="", "date_end"="", "time_start"="", "time_end"="", "low_limit"=0, "high_limit"=0, "records"=[], "column_headers"=[], "column_widths"=[]}, "REPORT_CBATCH_all_info"={"batch_code"="", "records"=[], "record_statuses"=[], "column_headers"=[], "displayed_rows"=[], "displayed_statuses"=[], "column_widths"=[], "active_page"=0}, "REPORT_CMPNT_all_info"={"gear_serial"="", "records"=[], "column_headers"=[], "displayed_rows"=[], "column_widths"=[], "active_page"=0}, "REPORTS_references"={"front_panel_reference"=refnum, "SQL_listbox_reference"=refnum, "REPORT_page_first"=refnum, "REPORT_page_previous"=refnum, "REPORT_page_next"=refnum, "REPORT_page_last"=refnum, "REPORT_page_counter"=refnum, "REPORT_GEAR_serial"=refnum, "REPORT_GEAR_serial_display"=refnum, "REPORT_GEAR_station"=refnum, "REPORT_GEAR_header_data_display"=refnum, "REPORT_DATES_start"=refnum, "REPORT_DATES_end"=refnum, "REPORT_DATES_time_start"=refnum, "REPORT_DATES_time_end"=refnum, "REPORT_DATES_order_selection"=refnum, "REPORT_DATES_last_OP"=refnum, "REPORT_DATES_last_status"=refnum, "REPORT_PBATCH_batch_no"=refnum, "REPORT_PBATCH_order_selection"=refnum, "REPORT_PBATCH_last_op"=refnum, "REPORT_PBATCH_last_status"=refnum, "REPORT_OPRTN_operation"=refnum, "REPORT_OPRTN_start"=refnum, "REPORT_OPRTN_end"=refnum, "REPORT_OPRTN_time_start"=refnum, "REPORT_OPRTN_time_end"=refnum, "REPORT_OPRTN_order_selection"=refnum, "REPORT_OPRTN_last_status"=refnum, "REPORT_CFG_type"=refnum, "REPORT_CFG_start"=refnum, "REPORT_CFG_end"=refnum, "REPORT_CFG_time_start"=refnum, "REPORT_CFG_time_end"=refnum, "REPORT_CFG_order_selection"=refnum, "REPORT_CFG_op_filter"=refnum, "REPORT_AUDIT_start"=refnum, "REPORT_AUDIT_end"=refnum, "REPORT_AUDIT_time_start"=refnum, "REPORT_AUDIT_time_end"=refnum, "REPORT_AUDIT_order_selection"=refnum, "REPORT_AUDIT_op_filter"=refnum, "REPORT_AUDIT_status_filter"=refnum, "REPORT_OKNOK_start"=refnum, "REPORT_OKNOK_end"=refnum, "REPORT_OKNOK_time_start"=refnum, "REPORT_OKNOK_time_end"=refnum, "REPORT_REWORKS_start"=refnum, "REPORT_REWORKS_end"=refnum, "REPORT_REWORKS_time_start"=refnum, "REPORT_REWORKS_time_end"=refnum, "REPORT_REWORKS_from_OP"=refnum, "REPORT_REWORKS_to_OP"=refnum, "REPORT_REWORKS_order_selection"=refnum, "REPORT_PACE_start"=refnum, "REPORT_PACE_end"=refnum, "REPORT_PACE_time_start"=refnum, "REPORT_PACE_time_end"=refnum, "REPORT_PACE_low_limit"=refnum, "REPORT_PACE_high_limit"=refnum, "REPORT_CBATCH_batch_code"=refnum, "REPORT_CBATCH_order_selection"=refnum, "REPORT_CMPNT_gear_serial"=refnum}} ("REPORT_all_info"), "REPORTS_references"=w904) -> (w903:T2)
      }
    }
  }
  "error_out" <- w5
  "output" <- w1
